vi "Import.vi"(9 "warehosue database table":string[](array[string]), 10 "Path":path, 11 "connection in":T4) -> (3 "connection out":T4)   [LabVIEW 2017]
uses:
  <vilib>/addons/database/Connection.llb/Conn ObjectReference.ctl
  Control/item colum type.ctl
  Control/invoice colum type.ctl
  <vilib>/Utility/miscctls.llb/LVPointTypeDef.ctl
  <vilib>/Utility/miscctls.llb/LVRowAndColumnUnsignedTypeDef.ctl
  Control/State machine.ctl
  Control/Label data.ctl
  <vilib>/addons/database/Connection.llb/DB Tools Open Connec (Path).vi
  <vilib>/addons/_office/excel.llb/Excel Get Data ([str]).vi
  <vilib>/addons/database/Connection.llb/Conn Execute.vi
  <vilib>/addons/database/Recordset.llb/Rec Fetch Recordset Data (R).vi
  <vilib>/addons/database/Recordset.llb/Rec Destroy - Connection.vi
  <vilib>/addons/database/_DB Variant To Data/Database Variant To Data.xnode
  <vilib>/Utility/NIReport.llb/NI_report.lvclass
  <vilib>/addons/_office/NI_ReportGenerationToolkit.lvlib
  <vilib>/addons/database/NI_Database_API.lvlib
  <vilib>/Utility/NIReport.llb/Excel/NI_Excel.lvclass
panel:
  out "reference":refnum<vi>[](array[refnum])
  in  "Print Mode 2":bool=TRUE
  out "IQA":string
  out "stock":string
  in  "Print Mode":bool=TRUE
  in  "Print":bool
  in  "Item No.(F8)":i32
  in  "INVOICE_data":T1
  in  "item_data":T2
  out "item_data_name":string[](array[string])
  out "item_data_ctr":refnum<vi>[](array[refnum])
  out "WAREHOUSE":string
  out "ECODE":string
  out "INVOICE_data_ctr":refnum<vi>[](array[refnum])
  out "INVOICE_data_name":string[](array[string])
  out "File data":string[][](array[string])
  in  "Import data":T3 {"Import Date" format="%<%d/%m/%Y>T"}
  in  "Lot Maker (F9)":string
  in  "Location (F5)":string
  in  "Maker Code (F4)":string
  in  "BUTTON_ADD":bool
  in  "Quantity (F10)":string
  in  "Lot Size (F6)":string
  in  "Unit (F7)":string
  in  "Item Code (F3)":string
  in  "Part No (F2)":string(combo)
  in  "Barcode (F1)":string
  in  "Offset":string="0"
  in  "Length":string="0"
  in  "Maker":string(combo)
  in  "Part Name":string(combo)
  in  "Product":string(combo)
  out "Invoice Date":timestamp format="%<%d/%m/%Y>T"
  out "Invoice Code":string
  out "Table":string[][](table)
  # "INVOICE IMPORT"
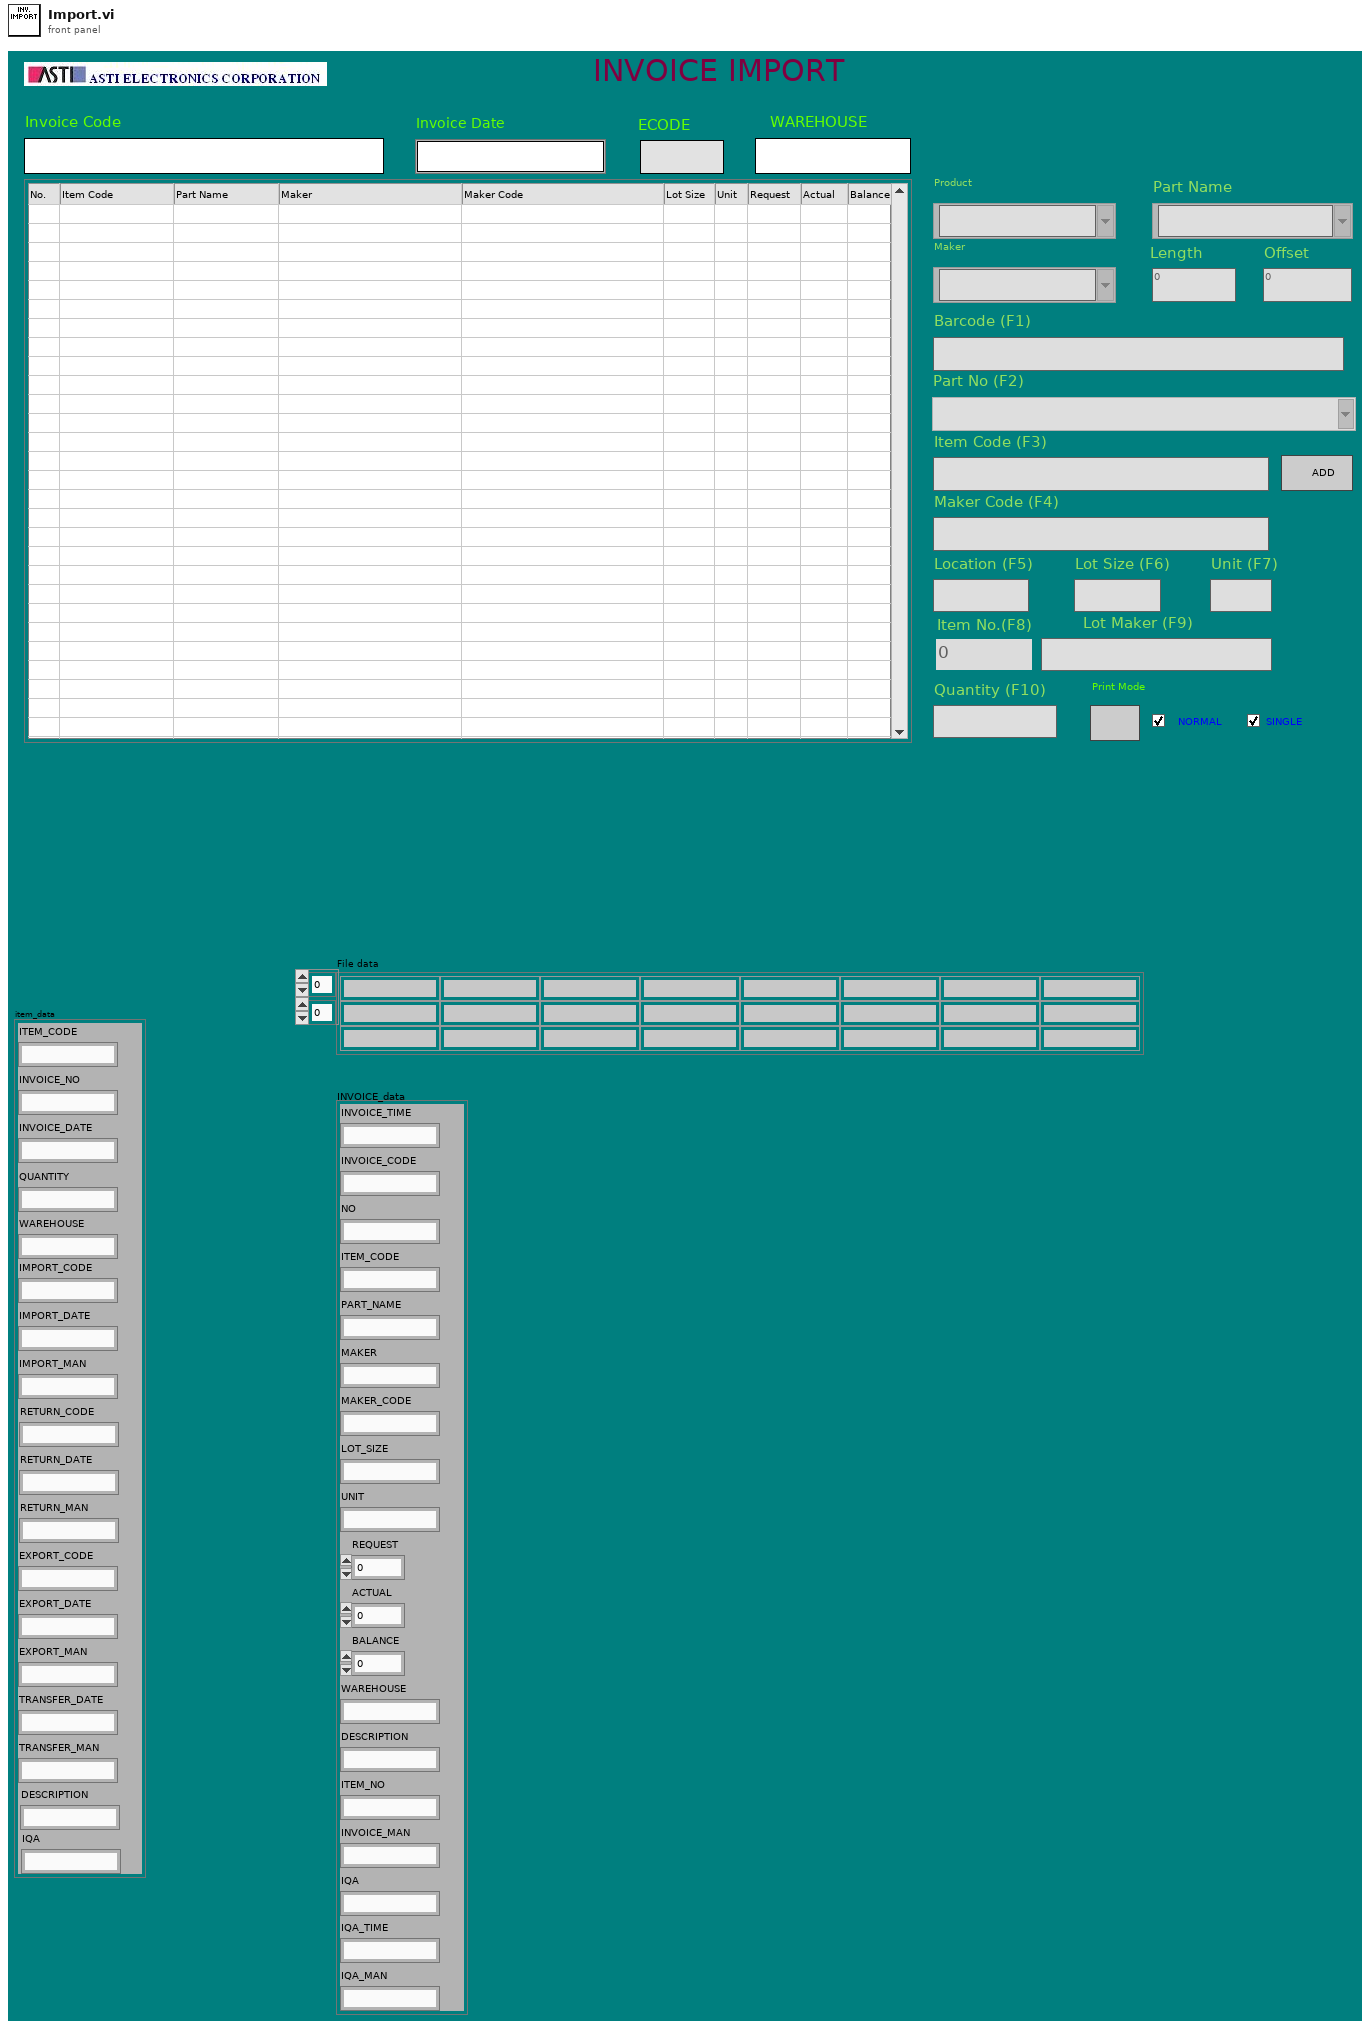
[diagram p1: front panel]
types:
  T1 = typedef "invoice colum type.ctl" = cluster{"INVOICE_TIME":string, "INVOICE_CODE":string, "NO":string, "ITEM_CODE":string, "PART_NAME":string, "MAKER":string, "MAKER_CODE":string, "LOT_SIZE":string, "UNIT":string, "REQUEST":dbl, "ACTUAL":dbl, "BALANCE":dbl, "WAREHOUSE":string, "DESCRIPTION":string, "ITEM_NO":string, "INVOICE_MAN":string, "IQA":string, "IQA_TIME":string, "IQA_MAN":string}
  T2 = typedef "item colum type.ctl" = cluster{"ITEM_CODE":string, "INVOICE_NO":string, "INVOICE_DATE":string, "QUANTITY":string, "IMPORT_CODE":string, "IMPORT_DATE":string, "IMPORT_MAN":string, "RETURN_CODE":string, "RETURN_DATE":string, "RETURN_MAN":string, "EXPORT_CODE":string, "EXPORT_DATE":string, "EXPORT_MAN":string, "TRANSFER_DATE":string, "TRANSFER_MAN":string, "DESCRIPTION":string, "IQA":string, "WAREHOUSE":string}
  T3 = cluster{"Import Code":string, "Import Date":timestamp, "Import data":string[][]}
  T4 = typedef "NI_Database_API.lvlib/Conn ObjectReference.ctl" = refnum<k1>
  T5 = typedef "State machine.ctl" = enum16{"Licence check", "Initial", "Log in", "Creat Config file", "Network setting", "Creat database 1", "Creat database 2", "Creat database 3", "Transfer", "Begin", "Exit"}
  T6 = typedef "LVRowAndColumnUnsignedTypeDef.ctl" = cluster{"Row":u32, "Column":u32}
  T7 = typedef "LVPointTypeDef.ctl" = cluster{"Horizontal":i16, "Vertical":i16}
  T8 = enum8{"Enabled", "Disabled", "Disabled and Grayed Out"}
  T9 = enum16{"Standard Report", "HTML", "Word", "Excel"}
  T10 = enum16{"maximized", "minimized", "normal", "no change"}
  T11 = typedef "Label data.ctl" = cluster{"Item Code":string, "ECode":string, "Part No.":string, "Maker":string, "Quantity":string, "Location":string, "Product":string, "Invoice No":string, "Invoice Date":string, "Lot maker":string, "Item No":string, "Unit":string}
  T12 = typedef "NI_Database_API.lvlib/Rec ObjectReference.ctl" = refnum<k1>
  T13 = cluster{"[0]":string, "[1]":string, "[2]":string, "[3]":string, "[4]":string, "[5]":string, "[6]":string, "[7]":string, "[8]":string, "[9]":string}
  T14 = cluster{"[0]":string, "[1]":string, "[2]":string, "[3]":string, "[4]":string, "[5]":string, "[6]":string, "[7]":string, "[8]":string, "[9]":string}[]
  T15 = typedef "ex-im colum type.ctl" = cluster{"INVOICE_TIME":string, "INVOICE_CODE":string, "NO":string, "ITEM_CODE":string, "PART_NAME":string, "MAKER":string, "MAKER_CODE":string, "LOT_SIZE":string, "UNIT":string, "REQUEST":dbl, "ACTUAL":dbl, "BALANCE":dbl, "WAREHOUSE":string, "DESCRIPTION":string, "ITEM_NO":string, "INVOICE_MAN":string, "IQA":string, "IQA_TIME":string, "IQA_MAN":string}
  T16 = cluster{"date/time string":string, "Import Code":string}
  T17 = cluster{"Product":string, "Item Code (F3)":string, "Part Name":string, "Maker":string, "Maker Code (F4)":string, "Lot Size (F6)":string, "Unit (F7)":string, string, string, "Location (F5)":string}
  T18 = cluster{"Quantity (F10)":string, "ECODE":string, "Invoice Code":string, "Item Code (F3)":string, "Lot Maker (F9)":string, "stock":string, "IQA":string, "WAREHOUSE":string}
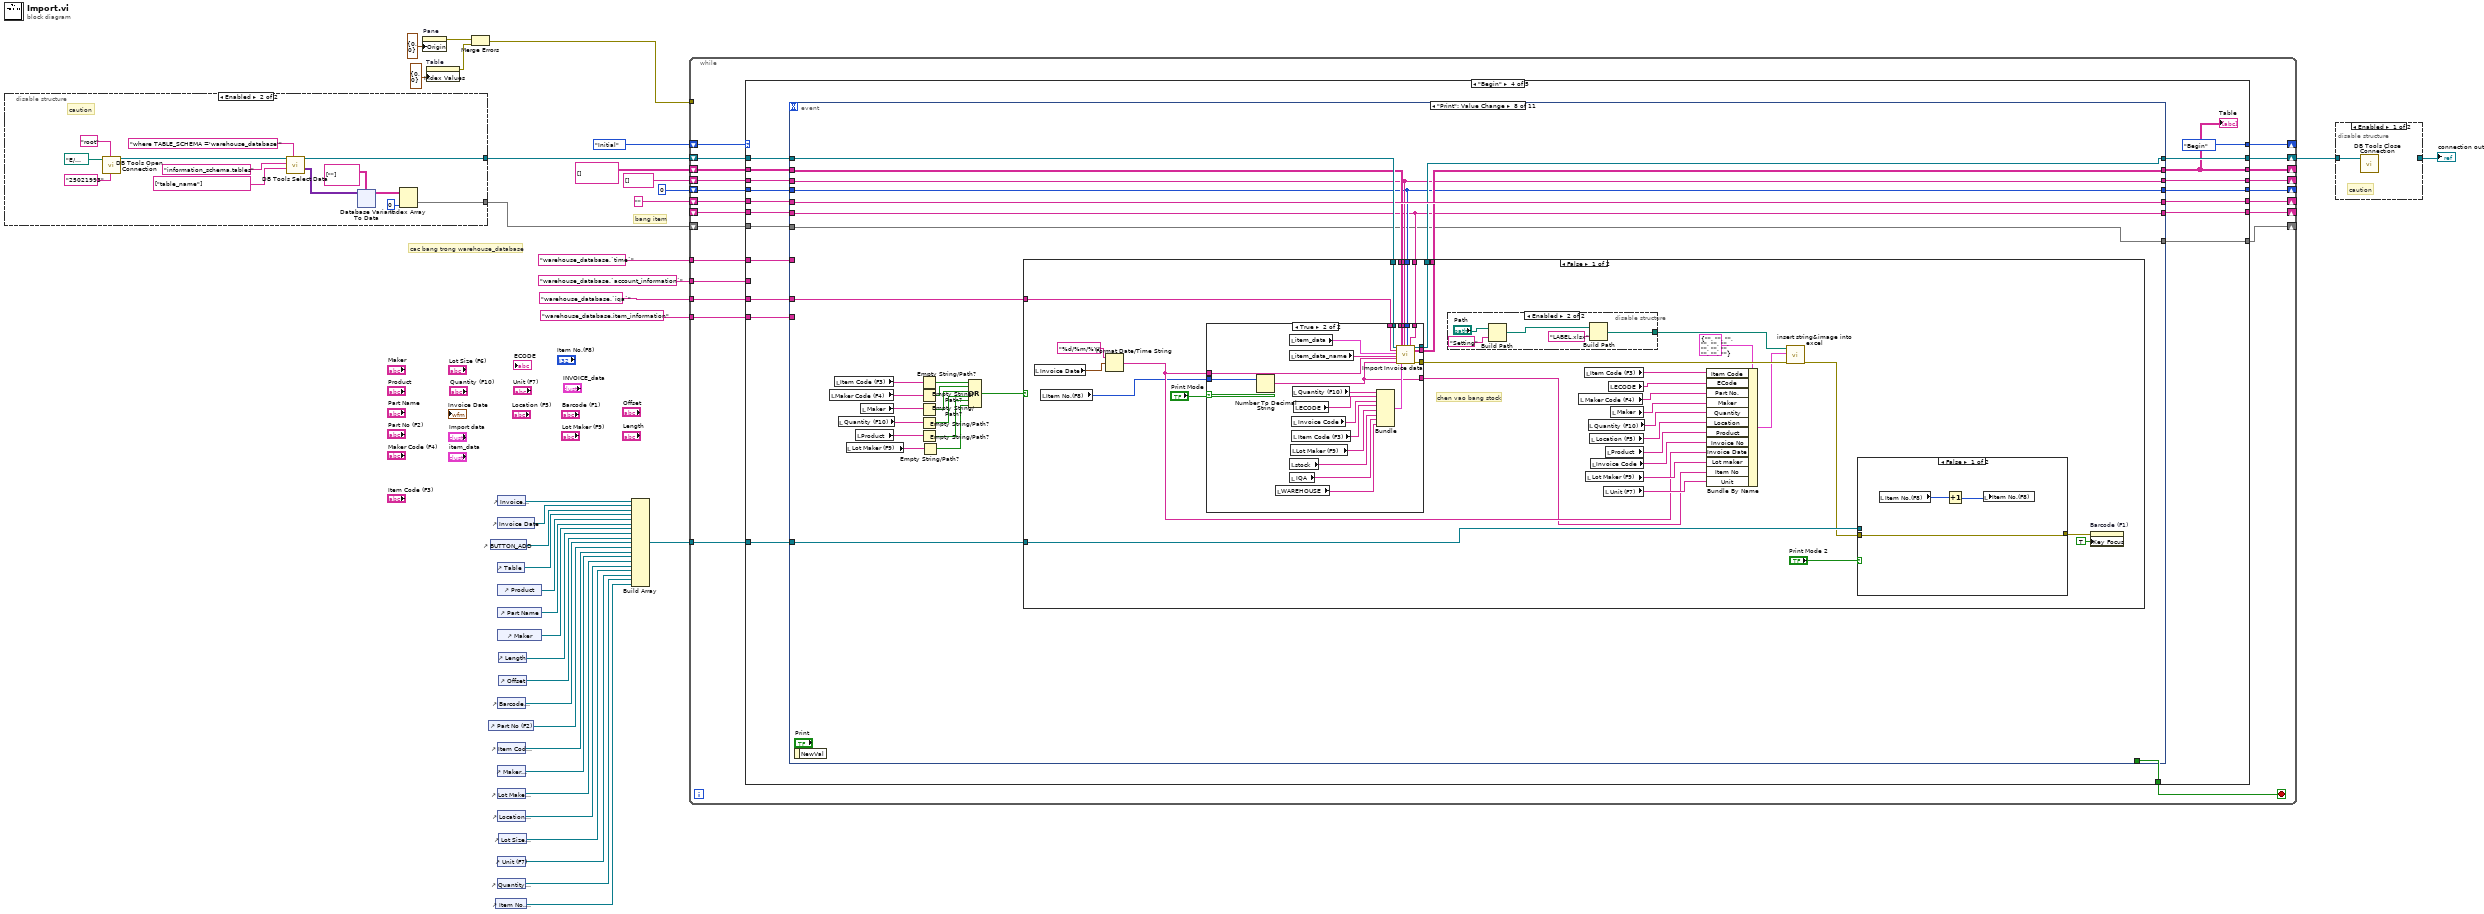
[diagram p0: block diagram]
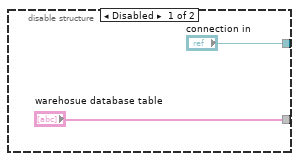
[diagram p3: hidden frame]
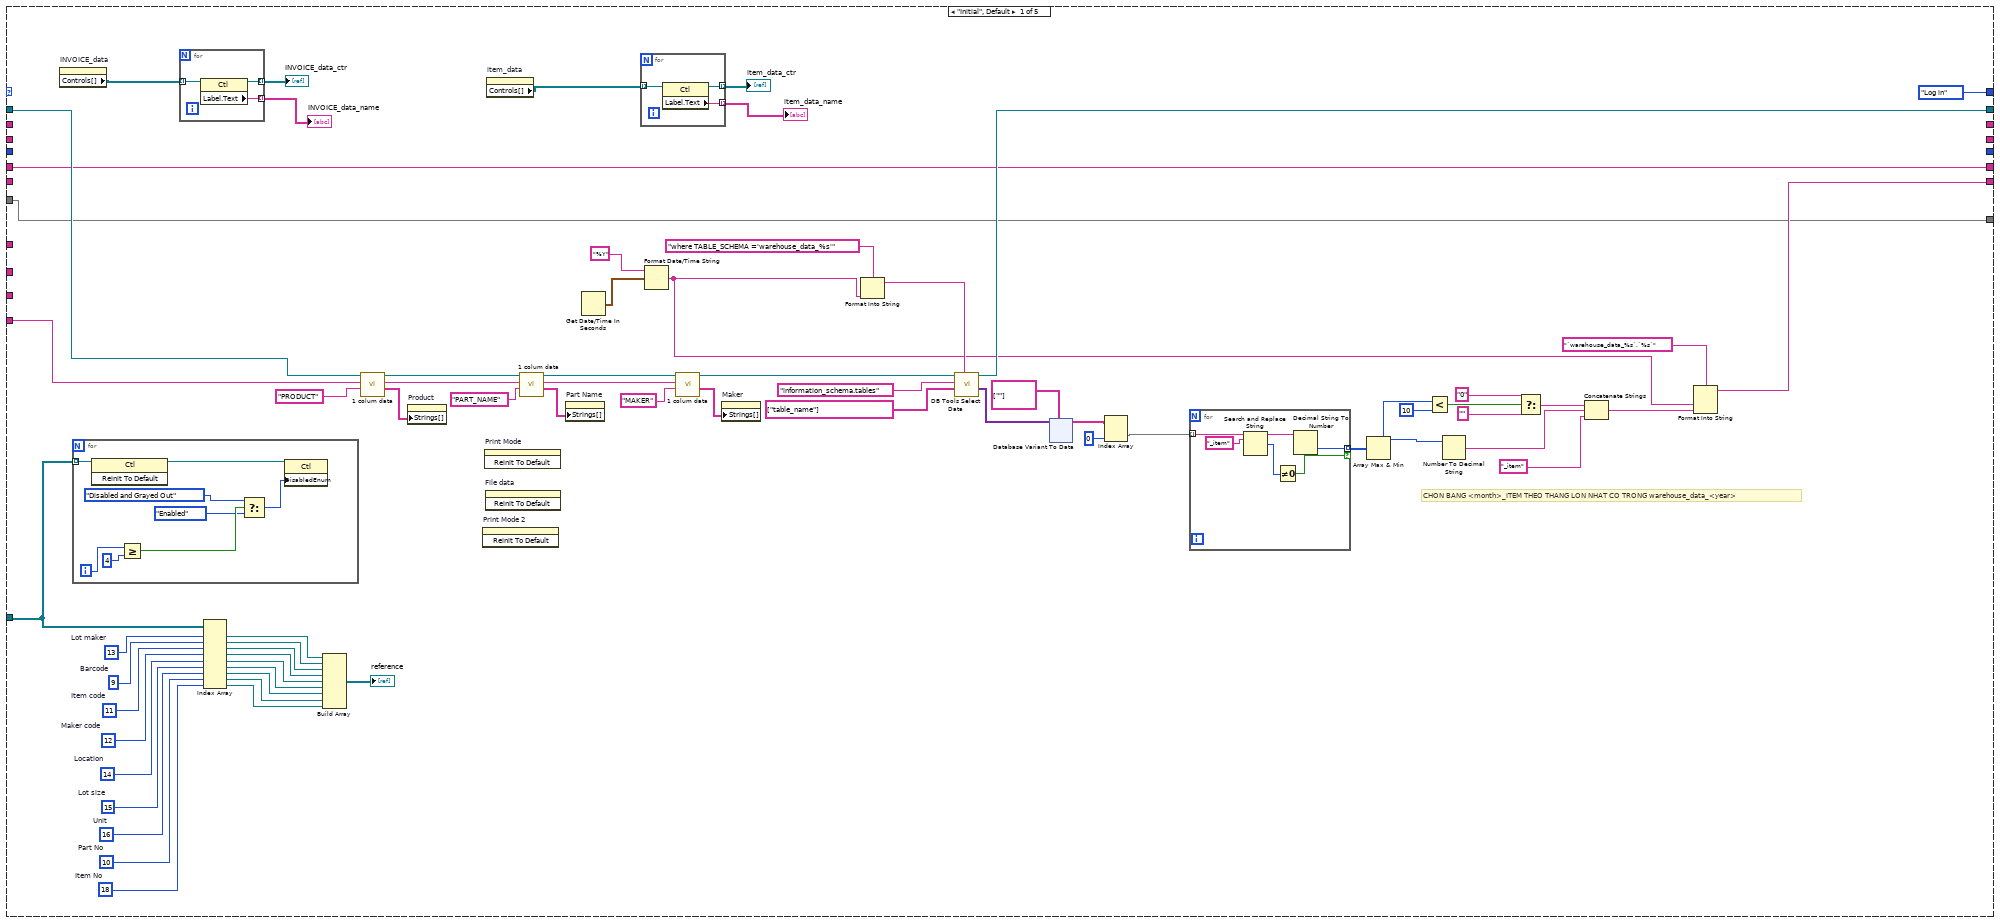
[diagram p4: hidden frame]
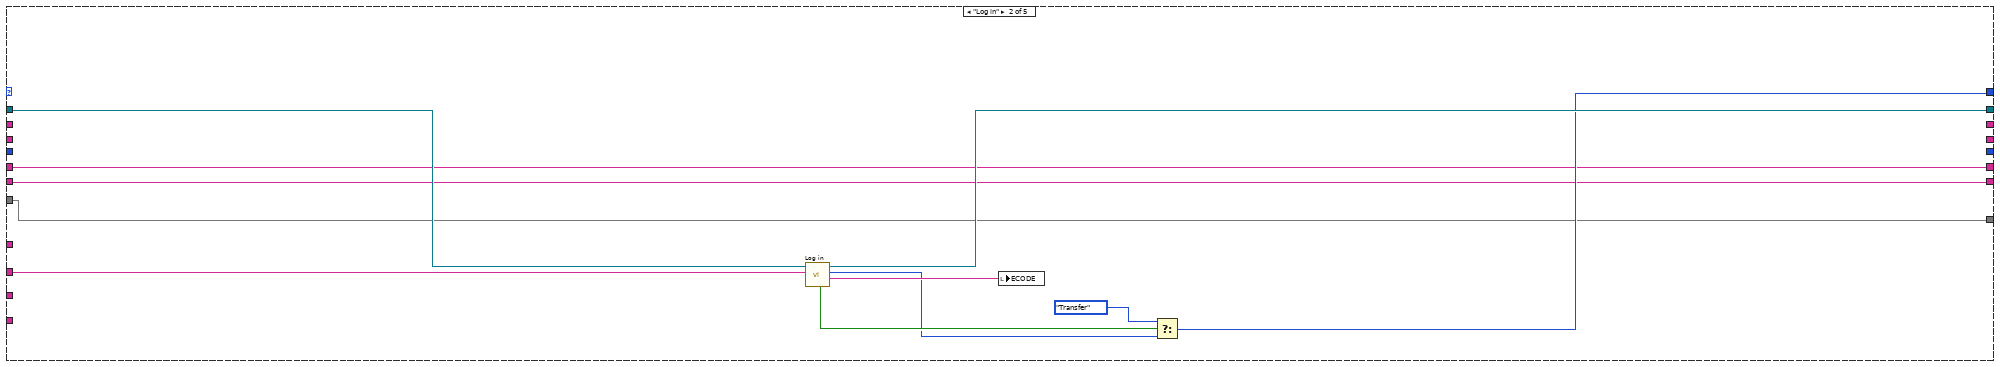
[diagram p5: hidden frame]
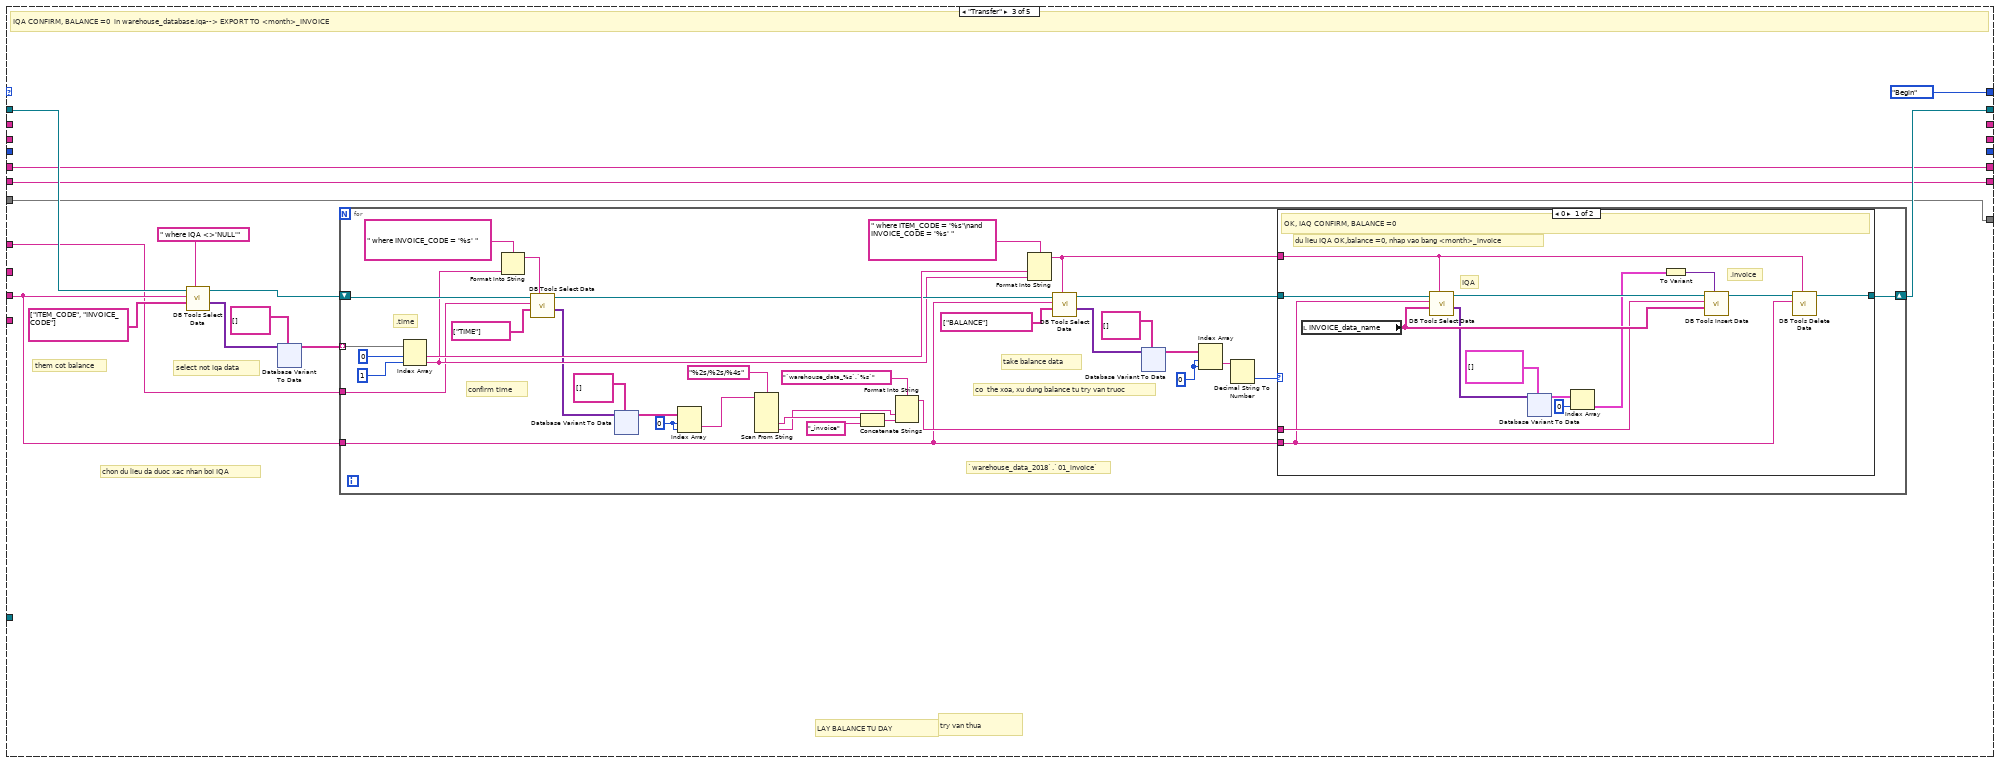
[diagram p6: hidden frame]
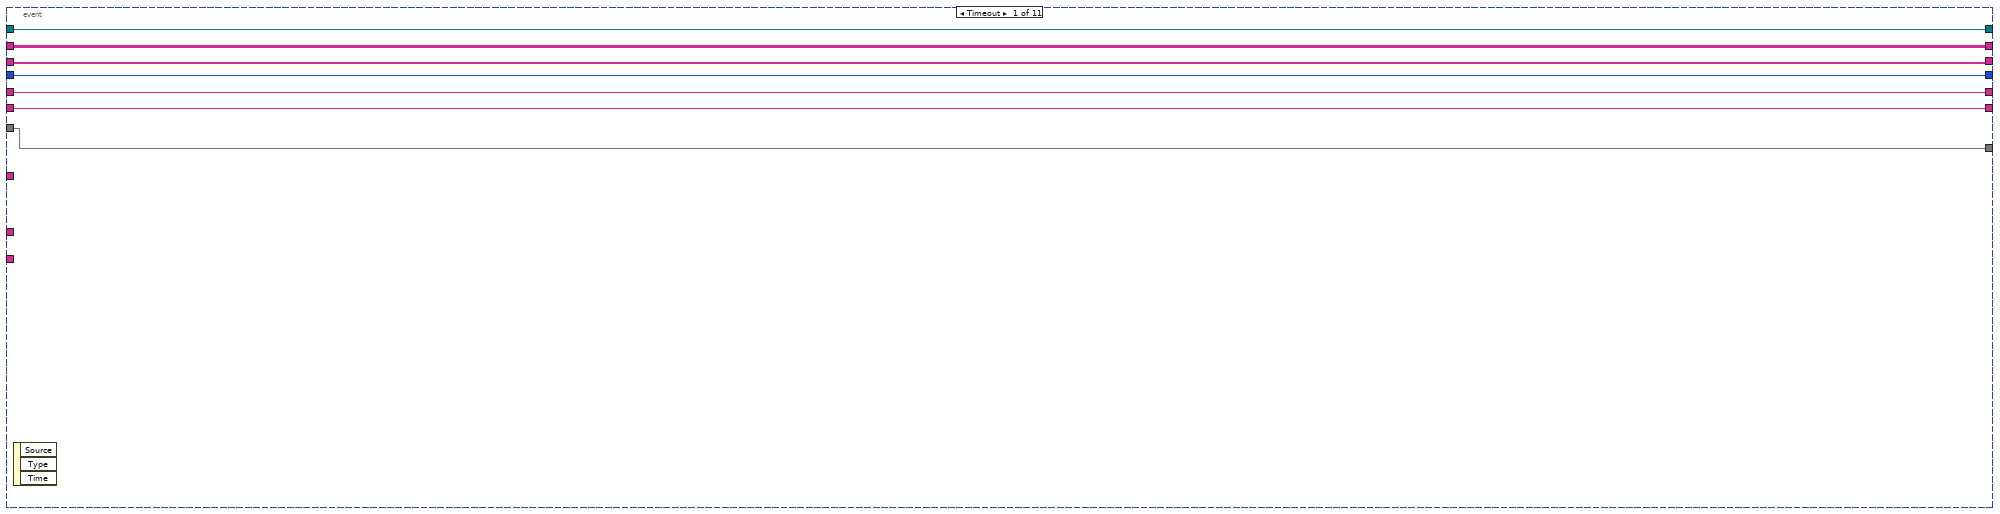
[diagram p8: hidden frame]
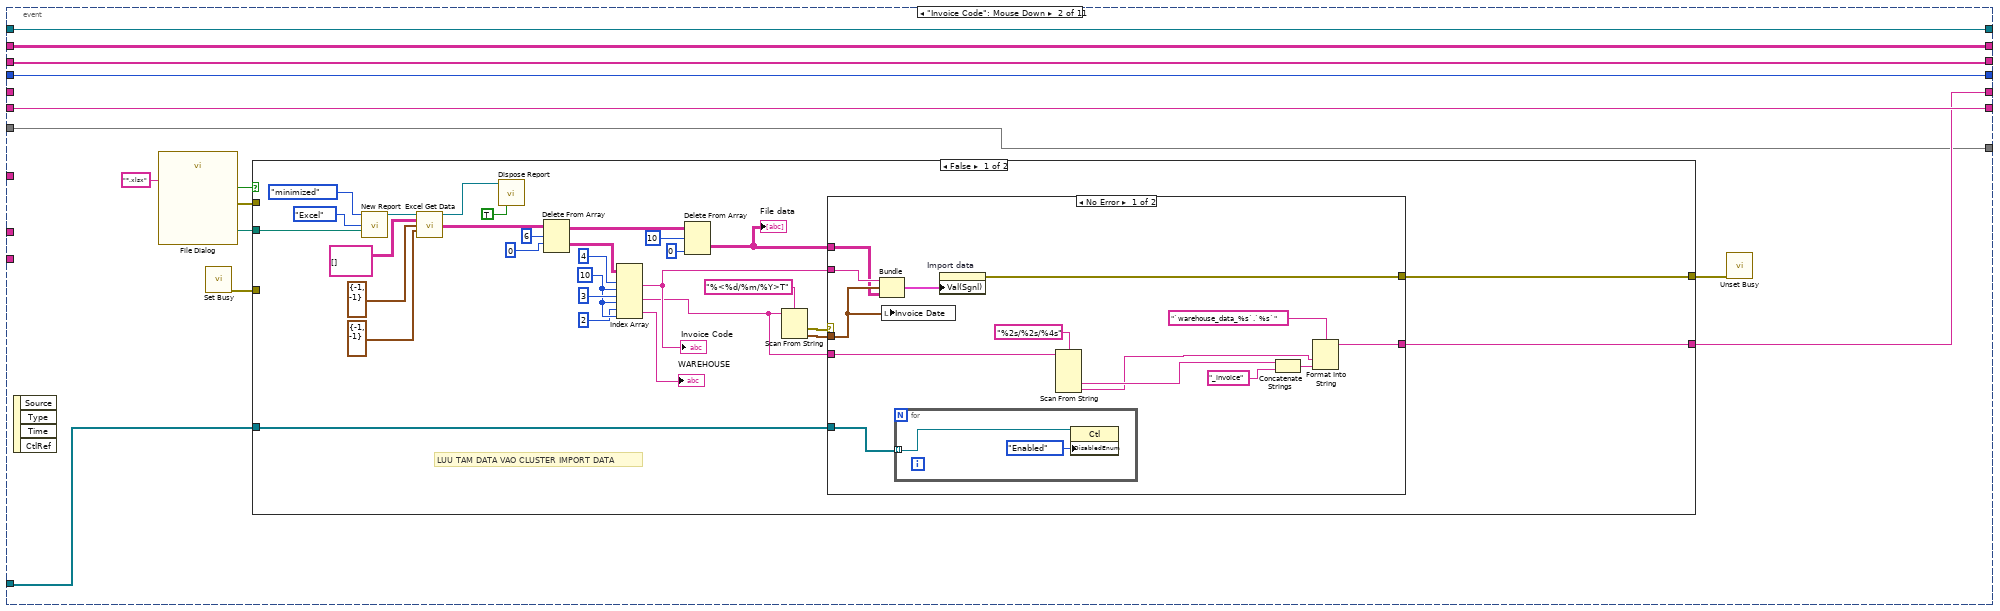
[diagram p9: hidden frame]
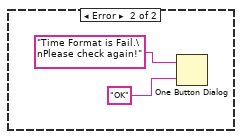
[diagram p10: hidden frame]
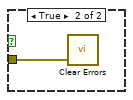
[diagram p11: hidden frame]
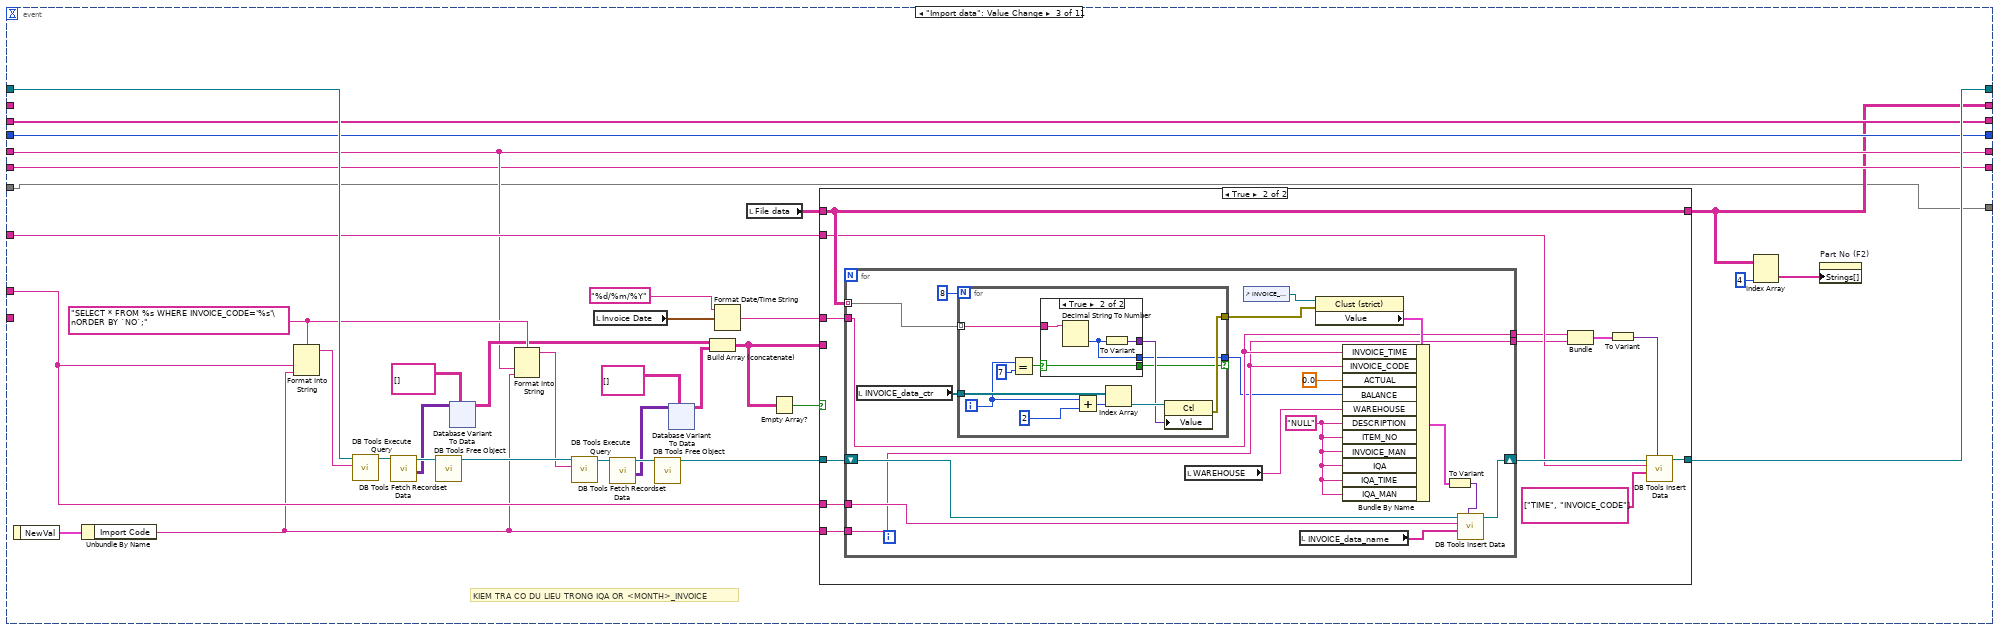
[diagram p12: hidden frame]
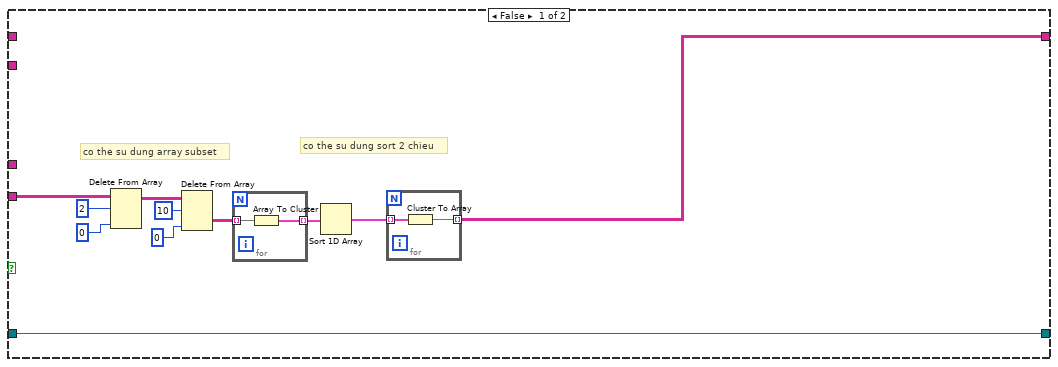
[diagram p13: hidden frame]
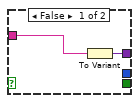
[diagram p14: hidden frame]
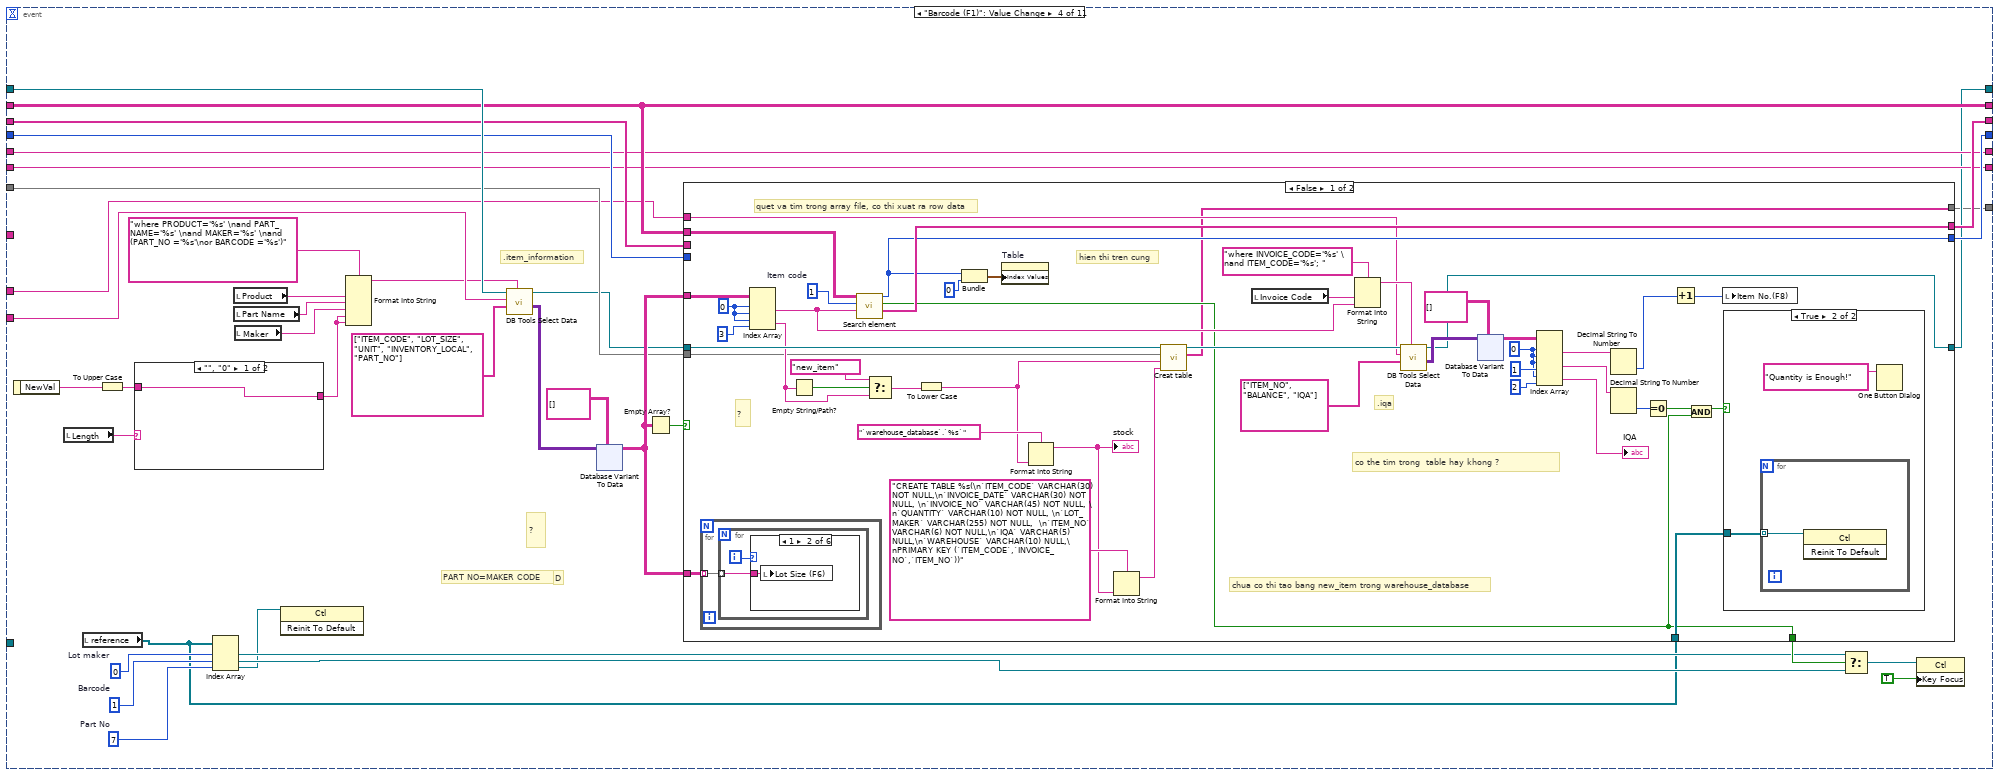
[diagram p15: hidden frame]
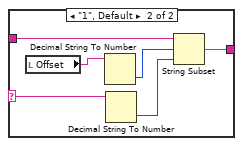
[diagram p16: hidden frame]
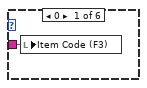
[diagram p18: hidden frame]
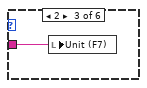
[diagram p19: hidden frame]
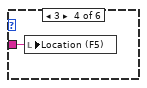
[diagram p20: hidden frame]
diagram:
  # "bang item"
  # "cac bang trong warehouse_database"
  n1 = disable-structure shown="Enabled" {
    disable-tunnel: ["connection in" w42] -> w16
    disable-tunnel: ["warehosue database table" w41] -> w3
    frame Disabled {
    }
    frame Enabled {
      # "caution"
      n2 = call-poly <vilib>:"DB Tools Open Connection.vi"("password"="25021993", "userID"="root", "connection information"=path "E:/PROJECT WORKING/23. WAREHOUSE/New Storage Management 2018/Setting/local.dsn") -> ("connection reference"=w43:T4)  [unwired: 5 in, 1 out]
      n3 = call <vilib>:"DB Tools Select Data.vi"("condition"="where TABLE_SCHEMA ='warehouse_database'", "columns"=string[] ["table_name"], "table"="information_schema.tables", "connection reference"=w43) -> ("data"=w46:variant[][], "connection reference out"=w42:T4)  [unwired: 2 in, 1 out]
      n4 = xnode "Database Variant To Data"("database variant"=w46, "type"=string[][] [[""]] ("columns")) -> ("data"=w48:string[][])  [unwired: 1 in, 1 out]
      n5 = Index Array(array=w48, index (col)=0 ("disabled index (col)")) -> (element=w41:string[])  [unwired: 1 in]
    }
  }
  n6 = property on="Pane" class="Pane"("Origin"=T7 {"Horizontal"=0, "Vertical"=0}) -> (error out=w36:errorcluster)  [unwired: 2 in, 1 out]
  n7 = property on="Table" class="Tbl (strict)"("Index Values"=T6 {"Row"=0, "Column"=0}) -> (error out=w35:errorcluster)  [unwired: 2 in, 1 out]
  n8 = Merge Errors(w36, w35) -> (w12:errorcluster)
  n9 = control-ref of="Part No (F2)"() -> (w25:refnum<vi>)
  n10 = control-ref of="BUTTON_ADD"() -> (w1:refnum<vi>)
  n11 = control-ref of="Item No.(F8)"() -> (w2:refnum<vi>)
  n12 = control-ref of="Invoice Code"() -> (w34:refnum<vi>)
  n13 = control-ref of="Invoice Date"() -> (w33:refnum<vi>)
  n14 = control-ref of="Table"() -> (w32:refnum<vi>)
  n15 = control-ref of="Product"() -> (w31:refnum<vi>)
  n16 = control-ref of="Part Name"() -> (w30:refnum<vi>)
  n17 = control-ref of="Maker"() -> (w29:refnum<vi>)
  n18 = control-ref of="Barcode (F1)"() -> (w26:refnum<vi>)
  n19 = control-ref of="Item Code (F3)"() -> (w24:refnum<vi>)
  n20 = control-ref of="Maker Code (F4)"() -> (w23:refnum<vi>)
  n21 = control-ref of="Lot Maker (F9)"() -> (w22:refnum<vi>)
  n22 = control-ref of="Location (F5)"() -> (w21:refnum<vi>)
  n23 = control-ref of="Unit (F7)"() -> (w19:refnum<vi>)
  n24 = control-ref of="Quantity (F10)"() -> (w13:refnum<vi>)
  n25 = control-ref of="Length"() -> (w28:refnum<vi>)
  n26 = control-ref of="Offset"() -> (w27:refnum<vi>)
  n27 = control-ref of="Lot Size (F6)"() -> (w20:refnum<vi>)
  n28 = Build Array(w34, w33, w1, w32, w31, w30, w29, w28, w27, w26, w25, w24, w23, w22, w21, w20, w19, w13, w2) -> (w18:refnum<vi>[])
  n29 = while {
    tunnel: w18 -> [w117]
    shift-right: [w116] -> _
    shift-left: State_machine."Initial" ("Enum") -> [w118]
    shift-right: [w114] -> w15
    shift-left: w16 -> [w115]
    tunnel: w12 -> [_]
    shift-right: [w113] -> _
    shift-left: string[][] [] ("File data") -> [w112]
    tunnel: "warehouse_database.item_information" -> [w110]
    shift-right: [w109] -> _
    shift-left: string[] [] ("row data") -> [w108]
    shift-right: [w107] -> _
    shift-left: 0 ("index") -> [w106]
    tunnel: "warehouse_database.`iqa`" -> [w105]
    tunnel: "warehouse_database.`account_information`" -> [w103]
    tunnel: "warehouse_database.`time`" -> [w102]
    shift-right: [w101] -> _
    shift-left: "" -> [w111]
    shift-right: [w100] -> _
    shift-left: _ -> [w104]
    shift-right: [w98] -> _
    shift-left: w3 -> [w99]
    stop <- w119 stop-if-true
    n30 = case shown="\"Begin\"" w118 {
      selector: w118 -> [_ _ _ _ w2042]
      tunnel: [_ _ _ w1076 TRUE ("T button?")] -> w119
      tunnel: w117 -> [w123 _ _ w1070 _]
      tunnel: [State_machine."Log in" ("Enum") w254 State_machine."Begin" ("Enum") State_machine."Begin" ("Enum") w2042] -> w116
      tunnel: w115 -> [w173 w261 w274 w1074 w2043]
      tunnel: [w162 w260 w266 w1073 w2043] -> w114
      tunnel: [_ _ _ w1072 _] -> w113
      tunnel: w112 -> [_ _ _ w1071 _]
      tunnel: w111 -> [w148 w252 w263 w1069 _]
      tunnel: w110 -> [w182 _ _ w1068 _]
      tunnel: [_ _ _ w1067 _] -> w109
      tunnel: w108 -> [_ _ _ w1066 _]
      tunnel: [_ _ _ w1065 _] -> w107
      tunnel: w106 -> [_ _ _ w1064 _]
      tunnel: w105 -> [_ _ w267 w1063 _]
      tunnel: w104 -> [_ w253 w265 w1062 w2041]
      tunnel: w103 -> [_ w259 _ _ _]
      tunnel: w102 -> [_ _ w264 w1061 _]
      tunnel: [w148 w252 w263 w1059 _] -> w101
      tunnel: [w149 w253 w265 w1060 w2041] -> w100
      tunnel: w99 -> [w120 w251 w262 w1058 w2040]
      tunnel: [w120 w251 w262 w1057 w2040] -> w98
      frame "Initial", Default {
        w127 = 18  # Item No
        w128 = 10  # Part No
        w135 = 16  # Unit
        w136 = 15  # Lot size
        w137 = 14  # Location
        w138 = 12  # Maker code
        w139 = 11  # Item code
        w140 = 9  # Barcode
        w141 = 13  # Lot maker
        # "CHON BANG <month>_ITEM THEO THANG LON NHAT CO TRONG warehouse_data_<year>"
        n31 = property on="INVOICE_data" class="Clust (strict)"() -> ("Controls[]"=w169:refnum<vi>[])  [unwired: 2 in, 2 out]
        n32 = for {
          tunnel: w123 -> [w250] mode=indexing
          i -> [w249]
          n33 = invoke class="Ctl" method="Reinit To Default"(reference=w250) -> (reference out=w247:refnum<vi>)  [unwired: 2 in, 2 out]
          n34 = Greater Or Equal?(x=w249, y=4) -> (x >= y?=w246:bool)
          n35 = Select(t=T8."Disabled and Grayed Out" ("Disabled"), s=w246, f=T8."Enabled" ("Disabled")) -> (s? t:f=w243:T8)
          n36 = property class="Ctl"(reference=w247, "DisabledEnum"=w243) -> ()  [unwired: 1 in, 2 out]
        }
        n37 = for {
          tunnel: w169 -> [w242] mode=indexing
          tunnel: [w241] -> w185 mode=indexing
          tunnel: [w240] -> w184 mode=indexing
          n38 = property class="Ctl"(reference=w242) -> (reference out=w240:refnum<vi>, "Label.Text"=w241:string)  [unwired: 1 in, 1 out]
        }
        "INVOICE_data_name" <- w185
        "INVOICE_data_ctr" <- w184
        n39 = Index Array(array=w123, index #1=w141, index #2=w140, index #3=w139, index #4=w138, index #5=w137, index #6=w136, index #7=w135, index #8=w128, index #9=w127) -> (element #1=w129:refnum<vi>, element #2=w124:refnum<vi>, element #3=w134:refnum<vi>, element #4=w133:refnum<vi>, element #5=w132:refnum<vi>, element #6=w131:refnum<vi>, element #7=w130:refnum<vi>, element #8=w125:refnum<vi>, element #9=w126:refnum<vi>)
        n40 = Build Array(w129, w124, w134, w133, w132, w131, w130, w125, w126) -> (→"reference":refnum<vi>[])
        n41 = call "1 colum data.vi"("column"="PRODUCT", "table"=w182, "Refnum in"=w173) -> ("data"=w180:string[], "table"=w179:string, "Refnum out"=w183:T4)  [unwired: 6 in]
        n42 = property on="Product" class="CmbBox"("Strings[]"=w180) -> ()  [unwired: 2 in, 2 out]
        n43 = invoke on="Print Mode 2" class="Bool (strict)" method="Reinit To Default"() -> ()  [unwired: 3 in, 3 out]
        n44 = invoke on="Print Mode" class="Bool (strict)" method="Reinit To Default"() -> ()  [unwired: 3 in, 3 out]
        n45 = invoke on="File data" class="Arr (strict)" method="Reinit To Default"() -> ()  [unwired: 3 in, 3 out]
        n46 = property on="item_data" class="Clust (strict)"() -> ("Controls[]"=w121:refnum<vi>[])  [unwired: 2 in, 2 out]
        n47 = call "1 colum data.vi"("column"="PART_NAME", "table"=w179, "Refnum in"=w183) -> ("data"=w177:string[], "table"=w172:string, "Refnum out"=w174:T4)  [unwired: 6 in]
        n48 = property on="Part Name" class="CmbBox"("Strings[]"=w177) -> ()  [unwired: 2 in, 2 out]
        n49 = Get Date/Time In Seconds() -> (seconds since 1Jan1904=w147:timestamp)
        n50 = for {
          tunnel: w121 -> [w239] mode=indexing
          tunnel: [w238] -> w170 mode=indexing
          tunnel: [w237] -> w171 mode=indexing
          n51 = property class="Ctl"(reference=w239) -> (reference out=w237:refnum<vi>, "Label.Text"=w238:string)  [unwired: 1 in, 1 out]
        }
        "item_data_name" <- w170
        "item_data_ctr" <- w171
        n52 = Format Date/Time String(time format string (%c)="%Y", seconds (now)=w147) -> (date/time string=w142:string)  [unwired: 1 in]
        n53 = call "1 colum data.vi"("column"="MAKER", "table"=w172, "Refnum in"=w174) -> ("data"=w176:string[], "Refnum out"=w163:T4)  [unwired: 6 in, 1 out]
        n54 = property on="Maker" class="CmbBox"("Strings[]"=w176) -> ()  [unwired: 2 in, 2 out]
        n55 = Format Into String(format string="where TABLE_SCHEMA ='warehouse_data_%s'" ("condition"), w142) -> (resulting string=w144:string)  [unwired: 2 in, 1 out]
        n56 = call <vilib>:"DB Tools Select Data.vi"("condition"=w144, "columns"=string[] ["table_name"], "table"="information_schema.tables", "connection reference"=w163) -> ("data"=w166:variant[][], "connection reference out"=w162:T4)  [unwired: 2 in, 1 out]
        n57 = xnode "Database Variant To Data"("database variant"=w166, "type"=string[][] [[""]] ("columns")) -> ("data"=w168:string[][])  [unwired: 1 in, 1 out]
        n58 = Index Array(array=w168, index (col)=0 ("disabled index (col)")) -> (element=w151:string[])  [unwired: 1 in]
        n59 = for {
          tunnel: w151 -> [w192] mode=indexing
          tunnel: [w187] -> w152 mode=indexing if=w189
          n60 = Search and Replace String(input string=w192, search string="_item") -> (result string=w188:string, number of replacements=w190:i32)  [unwired: 6 in, 2 out]
          n61 = Not Equal To 0?(x=w190) -> (x != 0?=w189:bool)
          n62 = Decimal String To Number(string=w188) -> (number=w187:i32)  [unwired: 2 in, 1 out]
        }
        n63 = Array Max & Min(array=w152) -> (max value=w153:i32)  [unwired: 3 out]
        n64 = Less?(x=w153, y=10) -> (x < y?=w155:bool)
        n65 = Number To Decimal String(number=w153) -> (decimal integer string=w159:string)  [unwired: 1 in]
        n66 = Select(t="0", s=w155, f="" ("t")) -> (s? t:f=w158:string)
        n67 = Concatenate Strings(w158, w159, "_item" ("string")) -> (w143:string)
        n68 = Format Into String(format string="`warehouse_data_%s`.`%s`", w142, w143) -> (resulting string=w149:string)  [unwired: 2 in, 1 out]
      }
      frame "Log in" {
        n69 = call "Log in.vi"("String in"=w259, "Refnum in"=w261) -> ("String out"=w258:string, "Enum"=w256:T5, "Refnum out"=w260:T4, "T/F"=w257:bool)  [unwired: 5 in, 1 out]
        n70 = local write "ECODE"(w258) -> ()
        n71 = Select(t=State_machine."Transfer", s=w257, f=w256) -> (s? t:f=w254:T5)
      }
      frame "Transfer" {
        # "LAY BALANCE TU DAY"
        # "try van thua"
        # "them cot balance"
        # "chon du lieu da duoc xac nhan boi IQA"
        # "select not iqa data"
        # "IQA CONFIRM, BALANCE =0  in warehouse_database.iqa--> EXPORT TO <month>_INVOICE"
        n72 = call <vilib>:"DB Tools Select Data.vi"("condition"=" where IQA <>'NULL'", "columns"=string[] ["ITEM_CODE", "INVOICE_CODE"], "table"=w267, "connection reference"=w274) -> ("data"=w271:variant[][], "connection reference out"=w268:T4)  [unwired: 2 in, 1 out]
        n73 = xnode "Database Variant To Data"("database variant"=w271, "type"=string[][] []) -> ("data"=w269:string[][])  [unwired: 1 in, 1 out]
        n74 = for {
          tunnel: w269 -> [w310] mode=indexing
          tunnel: w267 -> [w278]
          shift-right: [w297] -> w266
          shift-left: w268 -> [w307]
          tunnel: w264 -> [w290]
          w286 = 0 ("index (row)")
          w301 = 0 ("index (row)")
          # "co  the xoa, xu dung balance tu try van truoc"
          # "`warehouse_data_2018`.`01_invoice`"
          # ".time"
          # "take balance data"
          # "confirm time"
          n75 = Index Array(array=w310, index #1=0 ("index"), index #2=1 ("index")) -> (element #1=w305:string, element #2=w291:string)
          n76 = Format Into String(format string=" where INVOICE_CODE = '%s' " ("condition"), w291) -> (resulting string=w292:string)  [unwired: 2 in, 1 out]
          n77 = call <vilib>:"DB Tools Select Data.vi"("condition"=w292, "columns"=string[] ["TIME"], "table"=w290, "connection reference"=w307) -> ("data"=w287:variant[][], "connection reference out"=w294:T4)  [unwired: 2 in, 1 out]
          n78 = xnode "Database Variant To Data"("database variant"=w287, "type"=string[][] []) -> ("data"=w285:string[][])  [unwired: 1 in, 1 out]
          n79 = Index Array "Index Array"(array=w285, index (row)=w286, index (col)=w286) -> (element=w284:string)
          n80 = Scan From String(format string="%2s/%2s/%4s", input string=w284) -> (output 2=w280:string, output 3=w276:string)  [unwired: 6 in, 3 out]
          n81 = Concatenate Strings(w280, "_invoice" ("string")) -> (w277:string)
          n82 = Format Into String(format string="`warehouse_data_%s`.`%s`", w276, w277) -> (resulting string=w279:string)  [unwired: 2 in, 1 out]
          n83 = Format Into String(format string=" where ITEM_CODE = '%s'\nand INVOICE_CODE = '%s' " ("condition"), w305, w291) -> (resulting string=w295:string)  [unwired: 2 in, 1 out]
          n84 = call <vilib>:"DB Tools Select Data.vi"("condition"=w295, "columns"=string[] ["BALANCE"], "table"=w278, "connection reference"=w294) -> ("data"=w304:variant[][], "connection reference out"=w298:T4)  [unwired: 2 in, 1 out]
          n85 = xnode "Database Variant To Data"("database variant"=w304, "type"=string[][] []) -> ("data"=w302:string[][])  [unwired: 1 in, 1 out]
          n86 = Index Array(array=w302, index (row)=w301, index (col)=w301) -> (element=w300:string)
          n87 = Decimal String To Number(string=w300) -> (number=w299:i32)  [unwired: 2 in, 1 out]
          n88 = case shown="0" w299 {
            tunnel: w298 -> [w368 w968]
            tunnel: [w363 w968] -> w297
            tunnel: w278 -> [w362 _]
            tunnel: w279 -> [w365 _]
            tunnel: w295 -> [w361 _]
            frame 0 {
              # "du lieu IQA OK,balance =0, nhap vao bang <month>_invoice"
              # ".invoice"
              # "IQA"
              # "OK, IAQ CONFIRM, BALANCE =0"
              n89 = local read "INVOICE_data_name"() -> (w366:string[])
              n90 = call <vilib>:"DB Tools Select Data.vi"("condition"=w361, "columns"=w366, "table"=w362, "connection reference"=w368) -> ("data"=w360:variant[][], "connection reference out"=w367:T4)  [unwired: 2 in, 1 out]
              n91 = xnode "Database Variant To Data"("database variant"=w360, "type"=T1[] []) -> ("data"=w358:T1[])  [unwired: 1 in, 1 out]
              n92 = Index Array(array=w358, index=0) -> (element=w356:T1)
              n93 = To Variant(anything=w356) -> (Variant=w355:variant)
              n94 = call <vilib>:"DB Tools Insert Data.vi"("data"=w355, "columns"=w366, "table"=w365, "connection reference"=w367) -> ("connection reference out"=w364:T4)  [unwired: 6 in, 1 out]
              n95 = call <vilib>:"DB Tools Delete Data.vi"("condition"=w361, "table"=w362, "connection reference"=w364) -> ("connection reference out"=w363:T4)  [unwired: 7 in, 1 out]
            }
            frame 1, Default {
              # "khong lam gi ca"
            }
          }
        }
      }
      frame "Begin" {
        n96 = event shown="[7] \"Print\": Value Change" {
          selector: _ -> [_ _ _ _ _ _ _ _ _ _ _]
          dyn-events: _ -> [_ _ _ _ _ _ _ _ _ _ _]
          timeout: _ -> [_ _ _ _ _ _ _ _ _ _ _]
          tunnel: [_ _ _ _ _ _ _ _ _ _ w2038] -> w1076
          tunnel: w1074 -> [w1083 w1097 w1181 w1371 w1536 w1573 w1745 w1848 w1946 w2026 w2037]
          tunnel: [w1083 w1097 w1173 w1341 w1536 w1546 w1749 w1846 w1945 w2026 w2037] -> w1073
          tunnel: [w1082 w1095 w1150 w1353 w1535 w1557 w1748 w1844 w1944 w2025 w2036] -> w1072
          tunnel: w1071 -> [w1082 w1095 _ w1353 w1535 w1557 w1748 w1845 w1944 w2025 w2036]
          tunnel: w1070 -> [_ w1096 _ _ _ _ _ w1849 w1943 w2030 _]
          tunnel: w1069 -> [w1079 _ w1152 w1347 w1532 w1551 w1727 w1847 w1940 w2022 w2033]
          tunnel: w1068 -> [_ _ _ w1357 _ w1561 w1743 _ w1936 _ _]
          tunnel: [w1081 w1094 w1172 w1351 w1534 w1555 w1747 w1843 w1942 w2024 w2035] -> w1067
          tunnel: w1066 -> [w1081 w1094 w1172 w1350 w1534 w1554 w1747 w1843 w1942 w2024 w2035]
          tunnel: [w1080 w1093 w1171 w1349 w1533 w1553 w1746 w1842 w1941 w2023 w2034] -> w1065
          tunnel: w1064 -> [w1080 w1093 w1171 w1348 w1533 w1552 w1746 w1842 w1941 w2023 w2034]
          tunnel: w1063 -> [_ _ w1166 w1342 _ w1547 _ w1841 _ _ _]
          tunnel: w1062 -> [w1078 w1092 w1151 w1346 w1531 w1550 w1726 w1827 w1939 w2021 w2032]
          tunnel: w1061 -> [_ _ w1165 _ _ _ _ _ _ _ _]
          tunnel: [w1078 w1092 w1151 w1346 w1531 w1550 w1726 w1827 w1939 w2021 w2032] -> w1060
          tunnel: [w1079 w1091 w1152 w1347 w1532 w1551 w1727 w1847 w1940 w2022 w2033] -> w1059
          tunnel: w1058 -> [w1077 w1084 w1147 w1345 w1530 w1549 w1725 w1826 w1935 w2019 w2031]
          tunnel: [w1077 w1084 w1147 w1334 w1530 w1539 w1725 w1826 w1935 w2019 w2031] -> w1057
          event Timeout {
            n97 = event-data() -> ()  [unwired: 1 in, 3 out]
          }
          event "Invoice Code": Mouse Down {
            n98 = event-data() -> ()  [unwired: 1 in, 4 out]
            n99 = call "File Dialog"("pattern (all files)"="*.xlsx") -> ("selected path"=w1087:path, "cancelled"=w1089:bool, "error out"=w1088:errorcluster)  [unwired: 11 in, 1 out]
            n100 = call <vilib>:"Set Busy.vi"() -> ("error out"=w1086:errorcluster)  [unwired: 10 in, 1 out]
            n101 = case shown="False" w1089 {
              tunnel: w1088 -> [_ w1146]
              tunnel: w1087 -> [w1127 _]
              tunnel: w1086 -> [_ _]
              tunnel: [w1103 _] -> w1085
              tunnel: w1096 -> [w1104 _]
              tunnel: [w1101 _] -> w1091
              frame False {
                w1100 = 10 ("disabled index (col)")
                # "LUU TAM DATA VAO CLUSTER IMPORT DATA"
                n102 = call <vilib>:"New Report.vi"("window state (normal)"=T10."minimized", "report type"=T9."Excel", "template (empty)"=w1127) -> ("report out"=w1124:refnum<class "NI_report.lvclass">)  [unwired: 11 in, 1 out]
                n103 = call-poly <vilib>:"Excel Get Data.vi"("report in"=w1124, "data type"=string[][] [], "start (-1, -1)"=cluster{"start row":i32, "start column":i32} {"start row"=-1, "start column"=-1} ("start (0, 0)"), "end (-1, -1)"=cluster{"start row":i32, "start column":i32} {"start row"=-1, "start column"=-1} ("start (0, 0)")) -> ("report out"=w1123:refnum<class "NI_report.lvclass">, "data"=w1118:string[][])  [unwired: 9 in, 1 out]
                n104 = call-dynamic "Dispose Report.vi"("report in"=w1123, "close report? (T)"=TRUE) -> ()  [unwired: 13 in, 1 out]
                n105 = Delete From Array(array=w1118, length=6, index (row)=0 ("length")) -> (deleted portion=w1115:string[][], array with subset deleted=w1108:string[][])  [unwired: 1 in]
                n106 = Index Array(array=w1115, index (row) #1=4 ("index (row)"), index (col) #1=w1100, index (row) #2=3 ("disabled index (row)"), index (col) #2=w1100, index (row) #3=2 ("disabled index (row)"), index (col) #3=w1100) -> (element #1=w1109:string, element #2=w1102:string, element #3=→"WAREHOUSE":string)
                "Invoice Code" <- w1109
                n107 = Delete From Array(array=w1108, length=10, index (col)=0 ("disabled index (col)")) -> (deleted portion=w1105:string[][])  [unwired: 1 in, 1 out]
                "File data" <- w1105
                n108 = Scan From String(format string="%<%d/%m/%Y>T", input string=w1102) -> (error out=w1111:errorcluster, output 1=w1110:timestamp)  [unwired: 3 in, 2 out]
                n109 = case shown="No Error" w1111 {
                  tunnel: w1110 -> [w1139 _]
                  tunnel: w1105 -> [w1138 _]
                  tunnel: w1109 -> [w1140 _]
                  tunnel: w1104 -> [w1136 _]
                  tunnel: [w1137 _] -> w1103
                  tunnel: w1102 -> [w1135 _]
                  tunnel: [w1130 _] -> w1101
                  frame No Error {
                    n110 = Bundle(w1140, w1139, "data"=w1138) -> (w1141:cluster{string, timestamp, "data":string[][]})  [unwired: 1 in]
                    n111 = local write "Invoice Date"(w1139) -> ()
                    n112 = for {
                      tunnel: w1136 -> [w1143] mode=indexing
                      n113 = property class="Ctl"(reference=w1143, "DisabledEnum"=T8."Enabled" ("Disabled")) -> ()  [unwired: 1 in, 2 out]
                    }
                    n114 = property on="Import data" class="Clust (strict)"("Val(Sgnl)"=w1141) -> (error out=w1137:errorcluster)  [unwired: 2 in, 1 out]
                    n115 = Scan From String(format string="%2s/%2s/%4s", input string=w1135) -> (output 2=w1131:string, output 3=w1128:string)  [unwired: 6 in, 3 out]
                    n116 = Concatenate Strings(w1131, "_invoice" ("string")) -> (w1129:string)
                    n117 = Format Into String(format string="`warehouse_data_%s`.`%s`", w1128, w1129) -> (resulting string=w1130:string)  [unwired: 2 in, 1 out]
                  }
                  frame Error {
                    n118 = One Button Dialog(message="Time Format is Fail.\nPlease check again!", button name ("OK")="OK") -> ()  [unwired: 1 out]
                  }
                }
              }
              frame True {
                n119 = call <vilib>:"Clear Errors.vi"("error in (no error)"=w1146) -> ()  [unwired: 5 in, 2 out]
              }
            }
            n120 = call <vilib>:"Unset Busy.vi"("error in (no error)"=w1085) -> ()  [unwired: 10 in, 1 out]
          }
          event "Import data": Value Change {
            w1159 = "SELECT * FROM %s WHERE INVOICE_CODE='%s'\nORDER BY `NO`;"
            # "KIEM TRA CO DU LIEU TRONG IQA OR <MONTH>_INVOICE"
            n121 = event-data() -> ("NewVal"=w1180:T3)  [unwired: 1 in]
            n122 = Unbundle By Name(w1180) -> ("Import Code"=w1158:string)
            n123 = Format Into String(format string=w1159, w1166, w1158) -> (resulting string=w1179:string)  [unwired: 2 in, 1 out]
            n124 = call-poly <vilib>:"DB Tools Execute Query.vi"("SQL query"=w1179, "connection reference"=w1181) -> ("recordset reference"=w1178:T12)  [unwired: 6 in, 1 out]
            n125 = call-poly <vilib>:"DB Tools Fetch Recordset Data.vi"("recordset reference"=w1178) -> ("recordset data"=w1175:variant[][], "recordset reference out"=w1177:T12)  [unwired: 4 in, 1 out]
            n126 = call-poly <vilib>:"DB Tools Free Object.vi"("recordset reference"=w1177) -> ("connection reference"=w1160:T4)  [unwired: 9 in, 1 out]
            n127 = xnode "Database Variant To Data"("database variant"=w1175, "type"=string[][] []) -> ("data"=w1156:string[][])  [unwired: 1 in, 1 out]
            n128 = Format Into String(format string=w1159, w1152, w1158) -> (resulting string=w1157:string)  [unwired: 2 in, 1 out]
            n129 = call-poly <vilib>:"DB Tools Execute Query.vi"("SQL query"=w1157, "connection reference"=w1160) -> ("recordset reference"=w1164:T12)  [unwired: 6 in, 1 out]
            n130 = local read "Invoice Date"() -> (w1170:timestamp)
            n131 = call-poly <vilib>:"DB Tools Fetch Recordset Data.vi"("recordset reference"=w1164) -> ("recordset data"=w1161:variant[][], "recordset reference out"=w1163:T12)  [unwired: 4 in, 1 out]
            n132 = call-poly <vilib>:"DB Tools Free Object.vi"("recordset reference"=w1163) -> ("connection reference"=w1153:T4)  [unwired: 9 in, 1 out]
            n133 = xnode "Database Variant To Data"("database variant"=w1161, "type"=string[][] []) -> ("data"=w1155:string[][])  [unwired: 1 in, 1 out]
            n134 = Build Array (concatenate)(w1156, w1155) -> (w1154:string[][])
            n135 = Format Date/Time String(time format string (%c)="%d/%m/%Y", seconds (now)=w1170) -> (date/time string=w1169:string)  [unwired: 1 in]
            n136 = local read "File data"() -> (w1168:string[][])
            n137 = Empty Array?(array=w1154) -> (empty?=w1174:bool)
            n138 = case shown="True" w1174 {
              tunnel: [w1227 w1250] -> w1150
              tunnel: w1153 -> [w1231 w1253]
              tunnel: [w1231 w1247] -> w1173
              tunnel: w1158 -> [_ w1252]
              tunnel: w1154 -> [w1226 _]
              tunnel: w1169 -> [_ w1251]
              tunnel: w1168 -> [_ w1250]
              tunnel: w1166 -> [_ w1249]
              tunnel: w1165 -> [_ w1246]
              frame False {
                # "co the su dung sort 2 chieu"
                # "co the su dung array subset"
                n139 = Delete From Array "Delete From Array"(array=w1226, length=2, index (col)=0 ("disabled index (col)")) -> (array with subset deleted=w1234:string[][])  [unwired: 1 in, 1 out]
                n140 = Delete From Array(array=w1234, length=10, index (col)=0 ("disabled index (col)")) -> (deleted portion=w1230:string[][])  [unwired: 1 in, 1 out]
                n141 = for {
                  tunnel: w1230 -> [w1240] mode=indexing
                  tunnel: [w1239] -> w1229 mode=indexing
                  n142 = Array To Cluster(array=w1240) -> (cluster=w1239:T13)
                }
                n143 = Sort 1D Array(array=w1229) -> (sorted array=w1228:T14)
                n144 = for {
                  tunnel: w1228 -> [w1238] mode=indexing
                  tunnel: [w1237] -> w1227 mode=indexing
                  n145 = Cluster To Array(cluster=w1238) -> (array=w1237:string[])
                }
              }
              frame True {
                n146 = for {
                  shift-right: [w1270] -> w1248
                  shift-left: w1253 -> [w1271]
                  tunnel: w1250 -> [w1267] mode=indexing
                  tunnel: w1252 -> [w1255]
                  tunnel: w1251 -> [w1256]
                  tunnel: w1249 -> [w1259]
                  tunnel: [w1256] -> w1244
                  tunnel: [w1255] -> w1243
                  w1257 = "NULL" ("WAREHOUSE")
                  n147 = local read "INVOICE_data_ctr"() -> (w1266:refnum<vi>[])
                  n148 = for {
                    N: 8 -> [_]
                    tunnel: w1267 -> [w1276] mode=indexing
                    tunnel: w1266 -> [w1283]
                    tunnel: [w1274] -> w1265
                    tunnel: [w1273] -> w1254 if=w1272
                    i -> [w1279]
                    n149 = Equal?(x=w1279, y=7) -> (x = y?=w1277:bool)
                    n150 = case shown="True" w1277 {
                      selector: w1277 -> [_ w1286]
                      tunnel: w1276 -> [w1285 w1289]
                      tunnel: [w1284 w1288] -> w1275
                      tunnel: [_ w1287] -> w1273
                      tunnel: [_ w1286] -> w1272
                      frame False {
                        n151 = To Variant(anything=w1285) -> (Variant=w1284:variant)
                      }
                      frame True {
                        n152 = Decimal String To Number(string=w1289) -> (number=w1287:i32)  [unwired: 2 in, 1 out]
                        n153 = To Variant(anything=w1287) -> (Variant=w1288:variant)
                      }
                    }
                    n154 = Add(x=w1279, y=2) -> (x+y=w1281:i32)
                    n155 = Index Array(array=w1283, index=w1281) -> (element=w1280:refnum<vi>)
                    n156 = property class="Ctl"(reference=w1280, "Value"=w1275) -> (error out=w1274:errorcluster)  [unwired: 1 in, 1 out]
                  }
                  n157 = local read "WAREHOUSE"() -> (w1260:string)
                  n158 = control-ref of="INVOICE_data"() -> (w1258:refnum<vi>)
                  n159 = local read "INVOICE_data_name"() -> (w1268:string[])
                  n160 = property class="Clust (strict)"(reference=w1258, error in=w1265) -> ("Value"=w1264:T15)  [unwired: 2 out]
                  n161 = Bundle By Name(cluster=w1264, "INVOICE_TIME"=w1256, "INVOICE_CODE"=w1255, "ACTUAL"=0.0, "BALANCE"=w1254, "WAREHOUSE"=w1260, "DESCRIPTION"=w1257, "ITEM_NO"=w1257, "INVOICE_MAN"=w1257, "IQA"=w1257, "IQA_TIME"=w1257, "IQA_MAN"=w1257) -> (w1263:T15)
                  n162 = To Variant(anything=w1263) -> (Variant=w1269:variant)
                  n163 = call <vilib>:"DB Tools Insert Data.vi"("data"=w1269, "columns"=w1268, "table"=w1259, "connection reference"=w1271) -> ("connection reference out"=w1270:T4)  [unwired: 6 in, 1 out]
                }
                n164 = Bundle("date/time string"=w1244, "Import Code"=w1243) -> (w1242:T16)  [unwired: 1 in]
                n165 = To Variant(anything=w1242) -> (Variant=w1241:variant)
                n166 = call <vilib>:"DB Tools Insert Data.vi"("data"=w1241, "columns"=string[] ["TIME", "INVOICE_CODE"], "table"=w1246, "connection reference"=w1248) -> ("connection reference out"=w1247:T4)  [unwired: 6 in, 1 out]
              }
            }
            n167 = Index Array(array=w1150, index (col)=4 ("disabled index (col)")) -> (element=w1148:string[])  [unwired: 1 in]
            n168 = property on="Part No (F2)" class="CmbBox"("Strings[]"=w1148) -> ()  [unwired: 2 in, 2 out]
          }
          event "Barcode (F1)": Value Change {
            w1337 = 7  # Part No
            w1356 = 1  # Barcode
            w1359 = 0  # Lot maker
            # "?"
            # "D"
            # "PART NO=MAKER CODE"
            # ".item_information"
            n169 = event-data() -> ("NewVal"=w1365:string)  [unwired: 1 in]
            n170 = local read "Length"() -> (w1361:string)
            n171 = local read "reference"() -> (w1335:refnum<vi>[])
            n172 = To Upper Case(1:w1365) -> (0:w1360:string)
            n173 = case shown="\"\", \"0\"" w1361 {
              selector: w1361 -> [_ w1374]
              tunnel: w1360 -> [w1372 w1378]
              tunnel: [w1372 w1377] -> w1343
              frame "", "0" {
              }
              frame "1", Default {
                n174 = local read "Offset"() -> (w1376:string)
                n175 = Decimal String To Number(string=w1376) -> (number=w1375:i32)  [unwired: 2 in, 1 out]
                n176 = Decimal String To Number(string=w1374) -> (number=w1373:i32)  [unwired: 2 in, 1 out]
                n177 = String Subset(string=w1378, offset (0)=w1375, length (rest)=w1373) -> (substring=w1377:string)
              }
            }
            n178 = Index Array(array=w1335, index #1=w1359, index #2=w1356, index #3=w1337) -> (element #1=w1338:refnum<vi>, element #2=w1339:refnum<vi>, element #3=w1336:refnum<vi>)
            n179 = local read "Product"() -> (w1368:string)
            n180 = local read "Part Name"() -> (w1367:string)
            n181 = local read "Maker"() -> (w1366:string)
            n182 = invoke class="Ctl" method="Reinit To Default"(reference=w1336) -> ()  [unwired: 2 in, 3 out]
            n183 = Format Into String(format string="where PRODUCT='%s' \nand PART_NAME='%s' \nand MAKER='%s' \nand (PART_NO ='%s'\nor BARCODE ='%s')", w1368, w1367, w1366, w1343, w1343) -> (resulting string=w1340:string)  [unwired: 2 in, 1 out]
            n184 = call <vilib>:"DB Tools Select Data.vi"("condition"=w1340, "columns"=string[] ["ITEM_CODE", "LOT_SIZE", "UNIT", "INVENTORY_LOCAL", "PART_NO"], "table"=w1357, "connection reference"=w1371) -> ("data"=w1364:variant[][], "connection reference out"=w1344:T4)  [unwired: 2 in, 1 out]
            n185 = xnode "Database Variant To Data"("database variant"=w1364, "type"=string[][] []) -> ("data"=w1354:string[][])  [unwired: 1 in, 1 out]
            n186 = Empty Array?(array=w1354) -> (empty?=w1362:bool)
            n187 = case shown="False" w1362 {
              tunnel: w1354 -> [w1424 _]
              tunnel: [w1384 _] -> w1352
              tunnel: w1354 -> [w1420 _]
              tunnel: w1353 -> [w1419 _]
              tunnel: [w1418 w1483] -> w1351
              tunnel: w1350 -> [_ w1483]
              tunnel: [w1417 w1482] -> w1349
              tunnel: w1348 -> [_ w1482]
              tunnel: w1345 -> [w1382 w1480]
              tunnel: w1344 -> [w1416 w1481]
              tunnel: [w1380 w1481] -> w1341
              tunnel: w1342 -> [w1398 _]
              tunnel: w1335 -> [w1386 _]
              tunnel: [w1381 w1480] -> w1334
              frame False {
                w1390 = 0 ("index (row)")
                w1409 = 0 ("index (row)")
                w1423 = 1  # Item code
                # "?"
                # "hien thi tren cung"
                # "co the tim trong  table hay khong ?"
                # "quet va tim trong array file, co thi xuat ra row data"
                # ".iqa"
                # "chua co thi tao bang new_item trong warehouse_database"
                n188 = for {
                  tunnel: w1424 -> [w1472] mode=indexing
                  n189 = for {
                    tunnel: w1472 -> [w1473] mode=indexing
                    i -> [w1474]
                    n190 = case shown="1" w1474 {
                      tunnel: w1473 -> [w1475 w1476 w1477 w1478 w1479 _]
                      frame 0 {
                        n191 = local write "Item Code (F3)"(w1475) -> ()
                      }
                      frame 1 {
                        n192 = local write "Lot Size (F6)"(w1476) -> ()
                      }
                      frame 2 {
                        n193 = local write "Unit (F7)"(w1477) -> ()
                      }
                      frame 3 {
                        n194 = local write "Location (F5)"(w1478) -> ()
                      }
                      frame 4 {
                        n195 = local write "Maker Code (F4)"(w1479) -> ()
                      }
                      frame 5, Default {
                      }
                    }
                  }
                }
                n196 = Index Array(array=w1420, index (row) #1=w1409, index (col) #1=w1409, index (row) #2=w1409, index (col) #2=3 ("disabled index (col)")) -> (element #1=w1399:string, element #2=w1414:string)
                n197 = Empty String/Path?(string/path=w1414) -> (empty?=w1415:bool)
                n198 = call "Search element.vi"("element"=w1399, "Colum"=w1423, "all data"=w1419) -> ("row data"=w1418:string[], "Status"=w1384:bool, "index"=w1417:i32)  [unwired: 5 in, 1 out]
                n199 = Select(t="new_item", s=w1415, f=w1414) -> (s? t:f=w1406:string)
                n200 = To Lower Case(string=w1406) -> (all lower case string=w1405:string)
                n201 = Bundle("index"=w1417, 0) -> (w1421:cluster{"index":i32, i32})  [unwired: 1 in]
                n202 = property on="Table" class="Tbl (strict)"("Index Values"=w1421) -> ()  [unwired: 2 in, 2 out]
                n203 = Format Into String(format string="`warehouse_database`.`%s`", w1405) -> (resulting string=w1407:string)  [unwired: 2 in, 1 out]
                "stock" <- w1407
                n204 = Format Into String(format string="CREATE TABLE %s(\n`ITEM_CODE` VARCHAR(30) NOT NULL,\n`INVOICE_DATE` VARCHAR(30) NOT NULL, \n`INVOICE_NO` VARCHAR(45) NOT NULL, \n`QUANTITY` VARCHAR(10) NOT NULL, \n`LOT_MAKER` VARCHAR(255) NOT NULL,  \n`ITEM_NO` VARCHAR(6) NOT NULL,\n`IQA` VARCHAR(5) NULL,\n`WAREHOUSE` VARCHAR(10) NULL,\nPRIMARY KEY (`ITEM_CODE`,`INVOICE_NO`,`ITEM_NO`))", w1407) -> (resulting string=w1411:string)  [unwired: 2 in, 1 out]
                n205 = call "Creat table.vi"("query"=w1411, "table name"=w1405, "table data"=w1382, "Refnum in"=w1416) -> ("table data"=w1381:string[], "Refnum out"=w1400:T4)  [unwired: 6 in]
                n206 = local read "Invoice Code"() -> (w1404:string)
                n207 = Format Into String(format string="where INVOICE_CODE='%s' \nand ITEM_CODE='%s'; ", w1404, w1399) -> (resulting string=w1403:string)  [unwired: 2 in, 1 out]
                n208 = call <vilib>:"DB Tools Select Data.vi"("condition"=w1403, "columns"=string[] ["ITEM_NO", "BALANCE", "IQA"], "table"=w1398, "connection reference"=w1400) -> ("data"=w1387:variant[][], "connection reference out"=w1380:T4)  [unwired: 2 in, 1 out]
                n209 = xnode "Database Variant To Data"("database variant"=w1387, "type"=string[][] []) -> ("data"=w1396:string[][])  [unwired: 1 in, 1 out]
                n210 = Index Array(array=w1396, index (row) #1=w1390, index (col) #1=w1390, index (row) #2=w1390, index (col) #2=1 ("index (row)"), index (row) #3=w1390, index (col) #3=2 ("index (row)")) -> (element #1=w1395:string, element #2=w1393:string, element #3=→"IQA":string)
                n211 = Decimal String To Number(string=w1395) -> (number=w1383:i32)  [unwired: 2 in, 1 out]
                n212 = Decimal String To Number(string=w1393) -> (number=w1392:i32)  [unwired: 2 in, 1 out]
                n213 = Equal To 0?(x=w1392) -> (x = 0?=w1391:bool)
                n214 = Increment(x=w1383) -> (x+1=w1379:i32)
                n215 = And(x=w1391, y=w1384) -> (x .and. y?=w1385:bool)
                n216 = local write "Item No.(F8)"(w1379) -> ()
                n217 = case shown="True" w1385 {
                  tunnel: w1386 -> [_ w1425]
                  frame False {
                  }
                  frame True {
                    n218 = for {
                      tunnel: w1425 -> [w1427] mode=indexing
                      n219 = invoke class="Ctl" method="Reinit To Default"(reference=w1427) -> ()  [unwired: 2 in, 3 out]
                    }
                    n220 = One Button Dialog(message="Quantity is Enough!") -> ()  [unwired: 1 in, 1 out]
                  }
                }
              }
              frame True {
                n221 = One Button Dialog(message="THIS ITEM DON'T HAVE INFORMATION.\nPLEASE ADD INFORMATION !", button name ("OK")="OK") -> ()  [unwired: 1 out]
              }
            }
            n222 = Select(t=w1338, s=w1352, f=w1339) -> (s? t:f=w1355:refnum<vi>)
            n223 = property class="Ctl"(reference=w1355, "Key Focus"=TRUE) -> ()  [unwired: 1 in, 2 out]
          }
          event "Barcode (F1)", "Part No (F2)": Mouse Up {
            n224 = event-data() -> ()  [unwired: 1 in, 8 out]
            n225 = local read "reference"() -> (w1537:refnum<vi>[])
            n226 = for {
              tunnel: w1537 -> [w1538] mode=indexing
              n227 = invoke class="Ctl" method="Reinit To Default"(reference=w1538) -> ()  [unwired: 2 in, 3 out]
            }
          }
          event "Part No (F2)": Value Change {
            w1540 = 7  # Part No
            w1560 = 1  # Barcode
            w1563 = 0  # Lot maker
            n228 = event-data() -> ("NewVal"=w1567:string)  [unwired: 1 in]
            n229 = local read "reference"() -> (w1541:refnum<vi>[])
            n230 = To Upper Case(1:w1567) -> (0:w1543:string)
            n231 = local read "Product"() -> (w1570:string)
            n232 = local read "Part Name"() -> (w1569:string)
            n233 = local read "Maker"() -> (w1568:string)
            n234 = Index Array(array=w1541, index #1=w1563, index #2=w1560, index #3=w1540) -> (element #1=w1544:refnum<vi>, element #2=w1542:refnum<vi>)  [unwired: 1 out]
            n235 = Format Into String(format string="where PRODUCT='%s' \nand PART_NAME='%s' \nand MAKER='%s' \nand PART_NO ='%s'", w1570, w1569, w1568, w1543) -> (resulting string=w1545:string)  [unwired: 2 in, 1 out]
            n236 = invoke class="Ctl" method="Reinit To Default"(reference=w1542) -> ()  [unwired: 2 in, 3 out]
            n237 = call <vilib>:"DB Tools Select Data.vi"("condition"=w1545, "columns"=string[] ["ITEM_CODE", "LOT_SIZE", "UNIT", "INVENTORY_LOCAL", "PART_NO"], "table"=w1561, "connection reference"=w1573) -> ("data"=w1566:variant[][], "connection reference out"=w1548:T4)  [unwired: 2 in, 1 out]
            n238 = xnode "Database Variant To Data"("database variant"=w1566, "type"=string[][] []) -> ("data"=w1558:string[][])  [unwired: 1 in, 1 out]
            n239 = Empty Array?(array=w1558) -> (empty?=w1564:bool)
            n240 = case shown="False" w1564 {
              tunnel: w1558 -> [w1619 _]
              tunnel: [w1580 _] -> w1556
              tunnel: w1558 -> [w1615 _]
              tunnel: w1557 -> [w1614 _]
              tunnel: [w1613 w1678] -> w1555
              tunnel: w1554 -> [_ w1678]
              tunnel: [w1612 w1677] -> w1553
              tunnel: w1552 -> [_ w1677]
              tunnel: w1549 -> [w1575 w1675]
              tunnel: w1548 -> [w1611 w1676]
              tunnel: [w1582 w1676] -> w1546
              tunnel: w1547 -> [w1594 _]
              tunnel: w1541 -> [w1583 _]
              tunnel: [w1574 w1675] -> w1539
              frame False {
                w1586 = 0 ("index (row)")
                w1604 = 0 ("index (row)")
                w1618 = 1  # Item code
                # "? GIONG VOI BARCODE CHANGE VALUE"
                n241 = for {
                  tunnel: w1619 -> [w1667] mode=indexing
                  n242 = for {
                    tunnel: w1667 -> [w1668] mode=indexing
                    i -> [w1669]
                    n243 = case shown="4" w1669 {
                      tunnel: w1668 -> [w1670 w1671 w1672 w1673 w1674 _]
                      frame 0 {
                        n244 = local write "Item Code (F3)"(w1670) -> ()
                      }
                      frame 1 {
                        n245 = local write "Lot Size (F6)"(w1671) -> ()
                      }
                      frame 2 {
                        n246 = local write "Unit (F7)"(w1672) -> ()
                      }
                      frame 3 {
                        n247 = local write "Location (F5)"(w1673) -> ()
                      }
                      frame 4 {
                        n248 = local write "Maker Code (F4)"(w1674) -> ()
                      }
                      frame 5, Default {
                      }
                    }
                  }
                }
                n249 = Index Array(array=w1615, index (row) #1=w1604, index (col) #1=w1604, index (row) #2=w1604, index (col) #2=3 ("disabled index (col)")) -> (element #1=w1595:string, element #2=w1609:string)
                n250 = Empty String/Path?(string/path=w1609) -> (empty?=w1610:bool)
                n251 = call "Search element.vi"("element"=w1595, "Colum"=w1618, "all data"=w1614) -> ("row data"=w1613:string[], "Status"=w1580:bool, "index"=w1612:i32)  [unwired: 5 in, 1 out]
                n252 = Select(t="new_item", s=w1610, f=w1609) -> (s? t:f=w1602:string)
                n253 = To Lower Case(string=w1602) -> (all lower case string=w1601:string)
                n254 = Bundle("index"=w1612, 0) -> (w1616:cluster{"index":i32, i32})  [unwired: 1 in]
                n255 = property on="Table" class="Tbl (strict)"("Index Values"=w1616) -> ()  [unwired: 2 in, 2 out]
                n256 = Format Into String(format string="`warehouse_database`.`%s`", w1601) -> (resulting string=w1577:string)  [unwired: 2 in, 1 out]
                n257 = local write "stock"(w1577) -> ()
                n258 = Format Into String(format string="CREATE TABLE %s(\n`ITEM_CODE` VARCHAR(30) NOT NULL,\n`INVOICE_DATE` VARCHAR(30) NOT NULL, \n`INVOICE_NO` VARCHAR(45) NOT NULL, \n`QUANTITY` VARCHAR(10) NOT NULL, \n`LOT_MAKER` VARCHAR(255) NOT NULL,  \n`ITEM_NO` VARCHAR(6) NOT NULL,\n `IQA` VARCHAR(5) NULL,\n`WAREHOUSE` VARCHAR(10) NULL,\nPRIMARY KEY (`ITEM_CODE`,`INVOICE_NO`,`ITEM_NO`))", w1577) -> (resulting string=w1606:string)  [unwired: 2 in, 1 out]
                n259 = call "Creat table.vi"("query"=w1606, "table name"=w1601, "table data"=w1575, "Refnum in"=w1611) -> ("table data"=w1574:string[], "Refnum out"=w1596:T4)  [unwired: 6 in]
                n260 = local read "Invoice Code"() -> (w1600:string)
                n261 = Format Into String(format string="where INVOICE_CODE='%s' \nand ITEM_CODE='%s'; ", w1600, w1595) -> (resulting string=w1599:string)  [unwired: 2 in, 1 out]
                n262 = call <vilib>:"DB Tools Select Data.vi"("condition"=w1599, "columns"=string[] ["ITEM_NO", "BALANCE", "IQA"], "table"=w1594, "connection reference"=w1596) -> ("data"=w1584:variant[][], "connection reference out"=w1582:T4)  [unwired: 2 in, 1 out]
                n263 = xnode "Database Variant To Data"("database variant"=w1584, "type"=string[][] []) -> ("data"=w1592:string[][])  [unwired: 1 in, 1 out]
                n264 = Index Array(array=w1592, index (row) #1=w1586, index (col) #1=w1586, index (row) #2=w1586, index (col) #2=1 ("index (row)"), index (row) #3=w1586, index (col) #3=2 ("index (row)")) -> (element #1=w1591:string, element #2=w1589:string, element #3=w1578:string)
                n265 = local write "IQA"(w1578) -> ()
                n266 = Decimal String To Number(string=w1591) -> (number=w1579:i32)  [unwired: 2 in, 1 out]
                n267 = Decimal String To Number(string=w1589) -> (number=w1588:i32)  [unwired: 2 in, 1 out]
                n268 = Equal To 0?(x=w1588) -> (x = 0?=w1587:bool)
                n269 = Increment(x=w1579) -> (x+1=w1576:i32)
                n270 = And(x=w1587, y=w1580) -> (x .and. y?=w1581:bool)
                n271 = local write "Item No.(F8)"(w1576) -> ()
                n272 = case shown="True" w1581 {
                  tunnel: w1583 -> [_ w1620]
                  frame False {
                  }
                  frame True {
                    n273 = for {
                      tunnel: w1620 -> [w1622] mode=indexing
                      n274 = invoke class="Ctl" method="Reinit To Default"(reference=w1622) -> ()  [unwired: 2 in, 3 out]
                    }
                    n275 = One Button Dialog(message="Quantity is Enough!") -> ()  [unwired: 1 in, 1 out]
                  }
                }
              }
              frame True {
                n276 = One Button Dialog(message="THIS ITEM DON'T HAVE INFORMATION.\nPLEASE ADD INFORMATION !", button name ("OK")="OK") -> ()  [unwired: 1 out]
              }
            }
            n277 = Select(t=w1544, s=w1556, f=w1542) -> (s? t:f=w1559:refnum<vi>)
            n278 = property class="Ctl"(reference=w1559, "Key Focus"=TRUE) -> ()  [unwired: 1 in, 2 out]
          }
          event "BUTTON_ADD": Value Change {
            # ".item_information"
            n279 = event-data() -> ()  [unwired: 1 in, 1 out]
            n280 = local read "Item Code (F3)"() -> (w1740:string)
            n281 = local read "Length"() -> (w1731:string)
            n282 = local read "Offset"() -> (w1733:string)
            n283 = local read "Barcode (F1)"() -> (w1735:string)
            n284 = Format Into String(format string="where ITEM_CODE='%s';" ("condition"), w1740) -> (resulting string=w1728:string)  [unwired: 2 in, 1 out]
            n285 = To Upper Case(1:w1735) -> (0:w1732:string)
            n286 = call <vilib>:"DB Tools Select Data.vi"("condition"=w1728, "columns"=string[] ["PART_NO"], "table"=w1743, "connection reference"=w1745) -> ("data"=w1739:variant[][], "connection reference out"=w1744:T4)  [unwired: 2 in, 1 out]
            n287 = Concatenate Strings "Concatenate Strings"(w1731, "-" ("string"), w1733) -> (w1729:string)
            n288 = xnode "Database Variant To Data"("database variant"=w1739, "type"=string[][] []) -> ("data"=w1737:string[][])  [unwired: 1 in, 1 out]
            n289 = Empty Array?(array=w1737) -> (empty?=w1736:bool)
            n290 = case shown="\"\", \"0\"" w1731 {
              selector: w1731 -> [_ w1752]
              tunnel: w1732 -> [w1750 w1756]
              tunnel: [w1750 w1755] -> w1730
              frame "", "0" {
              }
              frame "1", Default {
                n291 = local read "Offset"() -> (w1754:string)
                n292 = Decimal String To Number(string=w1754) -> (number=w1753:i32)  [unwired: 2 in, 1 out]
                n293 = Decimal String To Number(string=w1752) -> (number=w1751:i32)  [unwired: 2 in, 1 out]
                n294 = String Subset(string=w1756, offset (0)=w1753, length (rest)=w1751) -> (substring=w1755:string)
              }
            }
            n295 = case shown="True" w1736 {
              tunnel: [w1757 w1780] -> w1749
              tunnel: w1744 -> [w1765 w1770]
              tunnel: w1743 -> [w1764 w1769]
              tunnel: w1740 -> [_ w1768]
              tunnel: w1730 -> [w1761 w1766]
              tunnel: w1729 -> [w1762 w1767]
              tunnel: w1728 -> [w1758 _]
              frame False {
                n296 = Bundle(w1762, w1761) -> (w1760:cluster{string, string})  [unwired: 1 in]
                n297 = To Variant(anything=w1760) -> (Variant=w1759:variant)
                n298 = call <vilib>:"DB Tools Update Data.vi"("condition"=w1758, "data"=w1759, "columns"=string[] ["`LENGTH-OFFSET`", "BARCODE"], "table"=w1764, "connection reference"=w1765) -> ("connection reference out"=w1757:T4)  [unwired: 5 in, 1 out]
              }
              frame True {
                # "THEM DU LIEU VAO BANG item_information"
                n299 = local read "Maker Code (F4)"() -> (w1775:string)
                n300 = local read "Lot Size (F6)"() -> (w1779:string)
                n301 = local read "Unit (F7)"() -> (w1774:string)
                n302 = local read "Location (F5)"() -> (w1773:string)
                n303 = local read "Part Name"() -> (w1777:string)
                n304 = local read "Maker"() -> (w1776:string)
                n305 = local read "Product"() -> (w1778:string)
                n306 = Bundle("Product"=w1778, "Item Code (F3)"=w1768, "Part Name"=w1777, "Maker"=w1776, "Maker Code (F4)"=w1775, "Lot Size (F6)"=w1779, "Unit (F7)"=w1774, w1767, w1766, "Location (F5)"=w1773) -> (w1772:T17)  [unwired: 1 in]
                n307 = To Variant(anything=w1772) -> (Variant=w1771:variant)
                n308 = call <vilib>:"DB Tools Insert Data.vi"("data"=w1771, "columns"=string[] ["PRODUCT", "ITEM_CODE", "PART_NAME", "MAKER", "PART_NO", "LOT_SIZE", "UNIT", "`LENGTH-OFFSET`", "BARCODE", "INVENTORY_LOCAL"], "table"=w1769, "connection reference"=w1770) -> ("connection reference out"=w1780:T4)  [unwired: 6 in, 1 out]
              }
            }
          }
          event "Print": Value Change {
            n309 = event-data() -> ()  [unwired: 1 in, 1 out]
            n310 = local read "Maker Code (F4)"() -> (w1839:string)
            n311 = local read "Item Code (F3)"() -> (w1840:string)
            n312 = local read "Quantity (F10)"() -> (w1837:string)
            n313 = local read "Lot Maker (F9)"() -> (w1829:string)
            n314 = local read "Product"() -> (w1836:string)
            n315 = local read "Maker"() -> (w1838:string)
            n316 = Empty String/Path?(string/path=w1840) -> (empty?=w1835:bool)
            n317 = Empty String/Path?(string/path=w1839) -> (empty?=w1834:bool)
            n318 = Empty String/Path?(string/path=w1838) -> (empty?=w1833:bool)
            n319 = Empty String/Path?(string/path=w1837) -> (empty?=w1832:bool)
            n320 = Empty String/Path?(string/path=w1836) -> (empty?=w1831:bool)
            n321 = Empty String/Path?(string/path=w1829) -> (empty?=w1828:bool)
            n322 = Compound Arithmetic op=OR(w1835, w1834, w1833, w1832, w1831, w1828) -> (w1830:bool)
            n323 = case shown="False" w1830 {
              tunnel: w1849 -> [w1881 _]
              tunnel: w1848 -> [w1879 w1934]
              tunnel: [w1867 w1934] -> w1846
              tunnel: w1845 -> [w1866 w1933]
              tunnel: [w1865 w1933] -> w1844
              tunnel: w1843 -> [w1864 _]
              tunnel: w1842 -> [w1863 _]
              tunnel: w1841 -> [w1861 _]
              tunnel: w1827 -> [w1856 _]
              frame False {
                # "chen vao bang stock"
                n324 = local read "Invoice Date"() -> (w1859:timestamp)
                n325 = local read "Item No.(F8)"() -> (w1854:i32)
                n326 = Format Date/Time String(time format string (%c)="%d/%m/%Y", seconds (now)=w1859) -> (date/time string=w1858:string)  [unwired: 1 in]
                n327 = case shown="True" "Print Mode" {
                  tunnel: w1879 -> [w1901 w1924]
                  tunnel: [w1901 w1918] -> w1867
                  tunnel: w1866 -> [w1900 w1917]
                  tunnel: [w1900 w1916] -> w1865
                  tunnel: w1864 -> [_ w1915]
                  tunnel: w1863 -> [_ w1914]
                  tunnel: [_ w1913] -> w1862
                  tunnel: w1861 -> [_ w1912]
                  tunnel: w1858 -> [_ w1908]
                  tunnel: w1854 -> [w1899 w1906]
                  tunnel: w1856 -> [_ w1907]
                  tunnel: [w1898 w1905] -> w1855
                  frame False {
                    n328 = Number To Decimal String(number=w1899) -> (decimal integer string=w1898:string)  [unwired: 1 in]
                  }
                  frame True {
                    n329 = Number To Decimal String(number=w1906) -> (decimal integer string=w1905:string)  [unwired: 1 in]
                    n330 = local read "WAREHOUSE"() -> (w1902:string)
                    n331 = local read "item_data"() -> (w1911:T2)
                    n332 = local read "item_data_name"() -> (w1910:string[])
                    n333 = local read "stock"() -> (w1904:string)
                    n334 = local read "IQA"() -> (w1903:string)
                    n335 = local read "Lot Maker (F9)"() -> (w1919:string)
                    n336 = local read "Invoice Code"() -> (w1921:string)
                    n337 = local read "Item Code (F3)"() -> (w1920:string)
                    n338 = local read "Quantity (F10)"() -> (w1923:string)
                    n339 = local read "ECODE"() -> (w1922:string)
                    n340 = Bundle("Quantity (F10)"=w1923, "ECODE"=w1922, "Invoice Code"=w1921, "Item Code (F3)"=w1920, "Lot Maker (F9)"=w1919, "stock"=w1904, "IQA"=w1903, "WAREHOUSE"=w1902) -> (w1909:T18)  [unwired: 1 in]
                    n341 = call "Import Invoice data.vi"("Refnum in"=w1924, "iqa"=w1912, "item_data"=w1911, "item_data_name"=w1910, "Invoive date"=w1908, "Item no"=w1905, "File data in"=w1917, "Import Data"=w1909, "row data"=w1915, "index"=w1914, "item"=w1907) -> ("Refnum out"=w1918:T4, "File data out"=w1916:string[][], "error out"=w1913:errorcluster)  [unwired: 6 in]
                  }
                }
                n342 = disable-structure shown="Enabled" {
                  disable-tunnel: [path "G:/06. Data/Data/05. AEC/07. New Storage Management/Setting/LABEL.xlsx" ("template (empty)") w1926] -> w1878
                  frame Disabled {
                    # "caution"
                  }
                  frame Enabled {
                    n343 = Build Path(base path="Path", name or relative path="Setting") -> (appended path=w1928:path)
                    n344 = Build Path(base path=w1928, name or relative path="LABEL.xlsx") -> (appended path=w1926:path)
                  }
                }
                n345 = local read "Maker Code (F4)"() -> (w1875:string)
                n346 = local read "Item Code (F3)"() -> (w1877:string)
                n347 = local read "Lot Maker (F9)"() -> (w1869:string)
                n348 = local read "Quantity (F10)"() -> (w1873:string)
                n349 = local read "Location (F5)"() -> (w1872:string)
                n350 = local read "Invoice Code"() -> (w1870:string)
                n351 = local read "Unit (F7)"() -> (w1868:string)
                n352 = local read "Product"() -> (w1871:string)
                n353 = local read "ECODE"() -> (w1876:string)
                n354 = local read "Maker"() -> (w1874:string)
                n355 = Bundle By Name(cluster=T11 {"Item Code"="", "ECode"="", "Part No."="", "Maker"="", "Quantity"="", "Location"="", "Product"="", "Invoice No"="", "Invoice Date"="", "Lot maker"="", "Item No"="", "Unit"=""} ("Item_Information"), "Item Code"=w1877, "ECode"=w1876, "Part No."=w1875, "Maker"=w1874, "Quantity"=w1873, "Location"=w1872, "Product"=w1871, "Invoice No"=w1870, "Invoice Date"=w1858, "Lot maker"=w1869, "Item No"=w1855, "Unit"=w1868) -> (w1852:T11)
                n356 = call "insert string&image into excel.vi"("error in"=w1862, "Item_Information"=w1852, "template Path"=w1878) -> ("error out"=w1851:errorcluster)  [unwired: 7 in, 1 out]
                n357 = case shown="False" "Print Mode 2" {
                  tunnel: w1881 -> [_ w1888]
                  tunnel: [w1885 w1887] -> w1880
                  tunnel: w1851 -> [w1885 w1886]
                  frame False {
                    n358 = local read "Item No.(F8)"() -> (w1884:i32)
                    n359 = Increment(x=w1884) -> (x+1=w1883:i32)
                    n360 = local write "Item No.(F8)"(w1883) -> ()
                  }
                  frame True {
                    n361 = for {
                      tunnel: w1888 -> [w1891] mode=indexing
                      tunnel: [w1890] -> w1887
                      tunnel: w1886 -> [w1889]
                      i -> [w1894]
                      n362 = Greater Or Equal?(x=w1894, y=9) -> (x >= y?=w1892:bool)
                      n363 = case shown="True" w1892 {
                        tunnel: w1891 -> [_ w1897]
                        tunnel: [_ w1896] -> w1890
                        tunnel: w1889 -> [_ w1895]
                        frame False {
                        }
                        frame True {
                          n364 = invoke class="Ctl" method="Reinit To Default"(reference=w1897, error in=w1895) -> (error out=w1896:errorcluster)  [unwired: 1 in, 2 out]
                        }
                      }
                    }
                  }
                }
                n365 = property on="Barcode (F1)" class="Str"(error in=w1880, "Key Focus"=TRUE) -> ()  [unwired: 1 in, 2 out]
              }
              frame True {
                n366 = One Button Dialog(message="Please check all information!\nITEM CODE\nMAKER CODE\nMAKER\nPRODUCT\nLOT MAKER\nQUANTITY", button name ("OK")="OK") -> ()  [unwired: 1 out]
              }
            }
          }
          event "Maker": Value Change {
            n367 = event-data() -> ("NewVal"=w1938:string)  [unwired: 1 in, 5 out]
            n368 = local read "Part Name"() -> (w1947:string)
            n369 = local read "Product"() -> (w1948:string)
            n370 = Empty String/Path?(string/path=w1948) -> (empty?=w1951:bool)
            n371 = Empty String/Path?(string/path=w1938) -> (empty?=w1937:bool)
            n372 = Empty String/Path?(string/path=w1947) -> (empty?=w1950:bool)
            n373 = Compound Arithmetic op=AND(w1951, w1950, w1937) -> (w1949:bool)
            n374 = case shown="False" w1949 {
              tunnel: w1938 -> [w1963 _]
              tunnel: w1948 -> [w1965 _]
              tunnel: w1947 -> [w1964 _]
              tunnel: w1946 -> [w1958 w2018]
              tunnel: [w1957 w2018] -> w1945
              tunnel: w1943 -> [w1956 _]
              tunnel: w1936 -> [w1952 _]
              frame False {
                w1955 = 9  # Barcode
                n375 = Index Array(array=w1956, index=w1955) -> (element=w1954:refnum<vi>)
                n376 = Format Into String(format string="where PRODUCT='%s'\n and PART_NAME='%s'\n and MAKER='%s'" ("condition"), w1965, w1964, w1963) -> (resulting string=w1973:string)  [unwired: 2 in, 1 out]
                n377 = property class="Ctl"(reference=w1954, "Key Focus"=TRUE) -> ()  [unwired: 1 in, 2 out]
                n378 = call <vilib>:"DB Tools Select Data.vi"("condition"=w1973, "columns"=string[] ["`LENGTH-OFFSET`"], "table"=w1952, "connection reference"=w1958) -> ("data"=w1967:variant[][], "connection reference out"=w1957:T4)  [unwired: 2 in, 1 out]
                n379 = xnode "Database Variant To Data"("database variant"=w1967, "type"=string[][] []) -> ("data"=w1969:string[][])  [unwired: 1 in, 1 out]
                n380 = Index Array(array=w1969, index (row)=0, index (col)=0 ("disabled index (col)")) -> (element=w1962:string)
                n381 = Match Pattern(string=w1962, regular expression="-") -> (before substring=w1960:string, after substring=w1959:string)  [unwired: 1 in, 2 out]
                n382 = local write "Offset"(w1959) -> ()
                n383 = local write "Length"(w1960) -> ()
              }
              frame True {
              }
            }
          }
          event "Lot Maker (F9)": Value Change {
            w2029 = 17  # Quantity
            n384 = event-data() -> ()  [unwired: 1 in, 6 out]
            n385 = local read "Lot Size (F6)"() -> (w2020:string)
            n386 = Index Array(array=w2030, index=w2029) -> (element=w2028:refnum<vi>)
            n387 = property class="Ctl"(reference=w2028, "Key Focus"=TRUE, "Value"=w2020) -> ()  [unwired: 1 in, 2 out]
          }
          event Panel Close? {
            n388 = event-data() -> ()  [unwired: 1 in, 4 out]
            n389 = call "Exit.vi"() -> ("T button?"=w2038:bool)  [unwired: 11 in]
            n390 = Not(x=w2038) -> (.not. x?=w2039:bool)
            n391 = event-data("Discard?"=w2039) -> ()  [unwired: 1 in, 1 out]
          }
        }
        "Table" <- w1072
      }
      frame "Exit" {
      }
    }
  }
  n392 = disable-structure shown="Enabled" {
    disable-tunnel: w15 -> [w2045 w2046]
    disable-tunnel: [_ w2046] -> w14
    frame Enabled {
      # "caution"
      n393 = call <vilib>:"DB Tools Close Connection.vi"("connection reference"=w2045) -> ()  [unwired: 6 in, 1 out]
    }
    frame Disabled {
    }
  }
  "connection out" <- w14
